vi "TF+Van der Pauw.vi"() -> ()   [LabVIEW 2022 SP3]
uses:
  <vilib>/Analysis/baseanly.llb/Mean (DBL).vi
  <vilib>/Utility/file.llb/Write Delimited Spreadsheet (DBL).vi
  <vilib>/Analysis/NI_AALBase.lvlib
panel:
  in  "FIxed F (Oe)":dbl format="%#_13g"
  out "Measured Field (Oe)":dbl=-0.24412487223744392
  out "Measured Temp (K)":dbl=2.0483396887779235
  in  "Ch2 Plot Clear":bool
  in  "Ch1 Plot Clear":bool
  out "Ch 1 phase":dbl=-151.82022434949218 caption="Ch1 phase" format="%.3p"
  out "Hall Voltage 1 phase":dbl=117.62016846841588 format="%.3p"
  out "Ch1 Current(mA)":dbl=0.0003122594054162884
  out "Hall Voltage1(mV)":dbl=0.015138421665849215
  in  "Fixed Field Approach":i32(ring) items=["Linear", "NoOvershoot", "Oscillate"]
  in  "Fixed F mode":i32(ring) items=["Persistent", "Driven"]
  in  "FIxed F Rate (Oe/s)":dbl=100.0 format="%#_13g"
  out "Hall Voltage 2 reletive phase":cluster{dbl[], dbl[]}(graph)={[0.09999999999999998, 0.12, 0.14, 0.16000000000000003, 0.17999999999999994, 0.19999999999999996, 0.21999999999999997, 0.24, 0.26, 0.28, 0.29999999999999993, 0.31999999999999995, 0.33999999999999997, 0.36, 0.38, 0.4, 0.42000000000000004, 0.43999999999999995, 0.45999999999999996, 0.48, 0.5, 0.52, 0.54, 0.56, 0.5800000000000001, 0.6, 0.62, 0.64, 0.6599999999999999, 0.6799999999999999, 0.7, 0.72, 0.74, 0.76, 0.78, 0.8, 0.8200000000000001, 0.84, 0.86, 0.88, 0.9, 0.92, 0.94, 0.96, 0.98, 1.0, 0.98, 0.96, 0.94, 0.92, 0.9, 0.88, 0.86, 0.84, 0.82, 0.8, 0.78, 0.76, 0.74, 0.72, 0.7, 0.6799999999999999, 0.66, 0.64, 0.62, 0.6, 0.58, 0.56, 0.54, 0.52, 0.5, 0.48, 0.45999999999999996, 0.44000000000000006, 0.42000000000000004, 0.4, 0.38, 0.36, 0.33999999999999997, 0.32, 0.30000000000000004, 0.28, 0.26, 0.24000000000000002, 0.22, 0.2, 0.18, 0.16, 0.14, 0.12000000000000001, 0.1, 0.09999999999999998, 0.12, 0.14, 0.16000000000000003, 0.17999999999999994, 0.19999999999999996, 0.21999999999999997, 0.24, 0.26, 0.28, 0.29999999999999993, 0.31999999999999995, 0.33999999999999997, 0.36, 0.38, 0.4, 0.42000000000000004, 0.43999999999999995, 0.45999999999999996, 0.48, 0.5, 0.52, 0.54, 0.56, 0.5800000000000001, 0.6, 0.62, 0.64, 0.6599999999999999, 0.6799999999999999, 0.7, 0.72, 0.74, 0.76, 0.78, 0.8, 0.8200000000000001, 0.84, 0.86, 0.88, 0.9, 0.92, 0.94, 0.96, 0.98, 1.0, 0.98, 0.96, 0.94, 0.92, 0.9, 0.88, 0.86, 0.84, 0.82, 0.8, 0.78, 0.76, 0.74, 0.72, 0.7, 0.6799999999999999, 0.66, 0.64, 0.62, 0.6, 0.58, 0.56, 0.54, 0.52, 0.5, 0.48, 0.45999999999999996, 0.44000000000000006, 0.42000000000000004, 0.4, 0.38, 0.36, 0.33999999999999997, 0.32, 0.30000000000000004, 0.28, 0.26, 0.24000000000000002, 0.22, 0.2, 0.18, 0.16, 0.14, 0.12000000000000001, 0.1], [117.62016846841588, 117.96664882272376, 118.35478696482726, 118.61912016643541, 118.76956664586604, 118.95054910823121, 119.01498123375443, 119.16872489157113, 119.24431424706378, 119.34190104277982, 119.41733225392822, 119.45140264855945, 119.53984114559682, 119.55691764422741, 119.59487520871042, 119.6750795139146, 119.68579169001923, 119.73065237331134, 119.74423324815396, 119.7661994334273, 119.80750346193834, 119.83623494650696, 119.82452268397942, 119.85627567058157, 119.86835371539776, 119.89360726965279, 119.90311700886441, 119.93603473890582, 119.94528450180692, 119.95000862999613, 119.95960465948625, 119.9830178122235, 119.97849406894788, 119.98959200475136, 119.99632464219606, 119.98257095958301, 120.01347012367368, 120.03103870555512, 120.04478039338926, 120.06360222149044, 120.05061637114048, 120.06363439063853, 120.07171311867637, 120.0757793318229, 120.09113199025303, 120.10726896331157, 120.06234962658894, 120.07718932923174, 120.09075423852748, 120.08476253619433, 120.05873660804704, 120.07529089338618, 120.07073006886651, 120.06602997484751, 120.06644594382928, 120.05437893498467, 120.0559832066358, 120.05241197254445, 120.03496471192462, 120.04190874507303, 120.04592984925304, 120.02590122679835, 120.02106762290221, 120.0170754772018, 120.01717601945583, 119.99024830583144, 119.98050754517847, 119.98548510957906, 119.96626810243879, 119.94421874372571, 119.91496186190318, 119.90254071057821, 119.89802448935203, 119.86225587700838, 119.84782030921231, 119.76071599522875, 119.78171218684165, 119.52712081973637, 119.68947818038498, 119.64888776868774, 119.54538024283588, 119.49187757183782, 119.40373568864177, 119.34094898550048, 119.25703379849283, 119.03268380413638, 118.93848534047406, 118.66368000738926, 118.3703709122756, 118.00894457485364, 117.8022869674905, 117.83191820734878, 118.35839994290589, 118.74306406859516, 118.97978381368443, 119.0832443256442, 119.22408053378842, 119.3756798875886, 119.42654507577663, 119.54312088447948, 119.65528936579355, 119.68067384348709, 119.73888591320637, 119.7746550722424, 119.83575660206921, 119.87436287491752, 119.92090575023776, 119.96360858392154, 119.97618916031327, 120.0270490763764, 120.03660757353578, 120.04594971613244, 120.07374861282088, 120.08502945701846, 120.11904718233538, 120.12373738373853, 120.13187955586031, 120.15078785675374, 120.16051712055169, 120.18138633972099, 120.18855573342282, 120.20283710115059, 120.21752926335739, 120.2286670939815, 120.25005622275296, 120.26083012867937, 120.26435687292016, 120.25219743715516, 120.27247788976976, 120.27728128431886, 120.30980987455453, 120.3013104315504, 120.30956542774932, 120.32575192936613, 120.32481345899741, 120.34376176879596, 120.32045496743885, 120.31980339045367, 120.31350527912403, 120.31252525198906, 120.3242014431218, 120.34462619894298, 120.32098729633576, 120.3242809008918, 120.31759933903815, 120.34279447419958, 120.29133105012681, 120.2971043007052, 120.2915107827317, 120.30887402170481, 120.3132908103599, 120.29180381456831, 120.29677581115975, 120.25488350003204, 120.25012405536286, 120.24749071884021, 120.20434065293489, 120.23689420155657, 120.20258149493482, 120.19465503125453, 120.16140368284456, 120.17158365673114, 120.12877813062116, 120.10707856478476, 120.07296661494834, 120.03335070293379, 120.02574871514983, 119.97110769112416, 120.18824358128647, 119.87610802993717, 119.85772779265321, 119.77209829112437, 119.73583766352138, 119.65849570448214, 119.57056721383769, 119.43100181965622, 119.2628284467831, 119.0562851102115, 118.80762144883226, 118.56712932086603, 117.71722366335914, 116.41351313841975, 116.41351313841975]}
  out "Hall Voltage 1 reletive phase":cluster{dbl[], dbl[]}(graph)={[0.09999999999999998, 0.12, 0.14, 0.16000000000000003, 0.17999999999999994, 0.19999999999999996, 0.21999999999999997, 0.24, 0.26, 0.28, 0.29999999999999993, 0.31999999999999995, 0.33999999999999997, 0.36, 0.38, 0.4, 0.42000000000000004, 0.43999999999999995, 0.45999999999999996, 0.48, 0.5, 0.52, 0.54, 0.56, 0.5800000000000001, 0.6, 0.62, 0.64, 0.6599999999999999, 0.6799999999999999, 0.7, 0.72, 0.74, 0.76, 0.78, 0.8, 0.8200000000000001, 0.84, 0.86, 0.88, 0.9, 0.92, 0.94, 0.96, 0.98, 1.0, 0.98, 0.96, 0.94, 0.92, 0.9, 0.88, 0.86, 0.84, 0.82, 0.8, 0.78, 0.76, 0.74, 0.72, 0.7, 0.6799999999999999, 0.66, 0.64, 0.62, 0.6, 0.58, 0.56, 0.54, 0.52, 0.5, 0.48, 0.45999999999999996, 0.44000000000000006, 0.42000000000000004, 0.4, 0.38, 0.36, 0.33999999999999997, 0.32, 0.30000000000000004, 0.28, 0.26, 0.24000000000000002, 0.22, 0.2, 0.18, 0.16, 0.14, 0.12000000000000001, 0.1, 0.09999999999999998, 0.12, 0.14, 0.16000000000000003, 0.17999999999999994, 0.19999999999999996, 0.21999999999999997, 0.24, 0.26, 0.28, 0.29999999999999993, 0.31999999999999995, 0.33999999999999997, 0.36, 0.38, 0.4, 0.42000000000000004, 0.43999999999999995, 0.45999999999999996, 0.48, 0.5, 0.52, 0.54, 0.56, 0.5800000000000001, 0.6, 0.62, 0.64, 0.6599999999999999, 0.6799999999999999, 0.7, 0.72, 0.74, 0.76, 0.78, 0.8, 0.8200000000000001, 0.84, 0.86, 0.88, 0.9, 0.92, 0.94, 0.96, 0.98, 1.0, 0.98, 0.96, 0.94, 0.92, 0.9, 0.88, 0.86, 0.84, 0.82, 0.8, 0.78, 0.76, 0.74, 0.72, 0.7, 0.6799999999999999, 0.66, 0.64, 0.62, 0.6, 0.58, 0.56, 0.54, 0.52, 0.5, 0.48, 0.45999999999999996, 0.44000000000000006, 0.42000000000000004, 0.4, 0.38, 0.36, 0.33999999999999997, 0.32, 0.30000000000000004, 0.28, 0.26, 0.24000000000000002, 0.22, 0.2, 0.18, 0.16, 0.14, 0.12000000000000001, 0.1], [-151.82022434949218, -151.31250474861076, -150.934829382567, -150.48587961112963, -150.35129794100732, -150.20108675684463, -150.07301012387398, -149.85371662190408, -149.80643007097768, -149.6778115966004, -149.70631232196195, -149.3427081876464, -144.00790971737905, -149.75303510022803, -149.67465048111166, -149.61059645892314, -149.5755216627079, -149.56032591732512, -149.56777135196236, -149.53038555798872, -149.4837567137922, -149.46653630858634, -149.4555130589029, -149.44977309701568, -149.46602213201024, -149.42050625632652, -149.44267585686146, -149.44000832559337, -149.42583379539636, -149.39692572431568, -149.40442155131146, -149.40915566881102, -149.38050614114596, -149.38240574949845, -149.3953243906204, -149.3899047221218, -149.38685008550175, -149.37072119411883, -149.37324923858517, -149.36914979835484, -149.37390639605138, -149.3980165878626, -149.38623806135408, -149.35518531108906, -149.37819742529774, -149.37025076997705, -149.37797439572273, -149.4274062049048, -149.39553532551332, -149.39989159256442, -149.40788326839706, -149.4035269042052, -149.42173829217444, -149.42516481564763, -149.4219167404996, -149.46356168834444, -149.4516805103338, -149.45047160544362, -149.45716135037998, -149.47450752769095, -149.4832252279336, -149.49183740199788, -149.51226639630787, -149.525555046651, -149.5573781565128, -149.5590093788641, -149.5858478680793, -149.5557150450339, -149.61888489114702, -149.65084954099694, -149.65437010384474, -149.69488018826033, -149.69116543387327, -149.7564704385459, -149.77576215560174, -149.78827998741025, -150.21783070990878, -156.94726445856756, -149.75208834187845, -149.79358735688876, -149.81920487838278, -149.97644416993913, -150.0531791626578, -150.16748042818656, -150.30076394633943, -150.44483707228213, -150.66626270081673, -151.04929447184827, -151.43411807203063, -151.97278023054187, -152.18821211537258, -152.14623356637654, -151.4719825276092, -150.96302427747355, -150.84756504567386, -150.5037700822142, -150.3245640418613, -150.17713325364664, -150.1036649225191, -149.99036753477975, -149.85697295444248, -149.8501754093205, -149.56080314237312, -146.67158122655187, -149.96749106410877, -149.93190810259412, -149.9232306144384, -149.8834345316244, -149.82170489643204, -149.7789775276986, -149.77872756893103, -149.7707527140453, -149.75157225999848, -149.7012296966859, -149.71638923850873, -149.69938903054089, -149.67312320269653, -149.69041977164406, -149.6838198853977, -149.66161778220618, -149.6546278866485, -149.640923821836, -149.6728863842432, -149.66791865505627, -149.62858582517933, -149.64183587402476, -149.6484558455101, -149.6427424788427, -149.6296817347956, -149.63395082883616, -149.62713187401155, -149.6182616601406, -149.65041315650092, -149.62494744989198, -149.61909696518853, -149.6175044512262, -149.6371509732279, -149.66137383135944, -149.63515614075328, -149.6451064613961, -149.65811060587708, -149.64909805431552, -149.6696824809014, -149.66829454461902, -149.65211834334818, -149.6792564836343, -149.69346020858046, -149.7169451406854, -149.71160254963883, -149.72665337378038, -149.73853617494782, -149.73020826238755, -149.75385526179556, -149.7724664962522, -149.77034769159013, -149.80481526391884, -149.81816596924764, -149.87205062927146, -149.86012342940273, -149.90891882509268, -149.92420949696478, -149.94160073513336, -149.98031714888242, -149.98297286567293, -150.01739729399605, -150.0978801191893, -150.09675943096, -149.9722562160305, -148.8947110005267, -150.0746278787694, -150.12829367372765, -150.21097166683603, -150.2349660580826, -150.3575760488762, -150.49529547074826, -150.72432289368865, -150.81632873807234, -151.05780214090098, -151.3722097867961, -151.68469888569936, -152.04933901054727, -152.04933901054727]}
  out "Hall Voltage 2":cluster{dbl[], dbl[]}(graph)={[0.09999999999999998, 0.12, 0.14, 0.16000000000000003, 0.17999999999999994, 0.19999999999999996, 0.21999999999999997, 0.24, 0.26, 0.28, 0.29999999999999993, 0.31999999999999995, 0.33999999999999997, 0.36, 0.38, 0.4, 0.42000000000000004, 0.43999999999999995, 0.45999999999999996, 0.48, 0.5, 0.52, 0.54, 0.56, 0.5800000000000001, 0.6, 0.62, 0.64, 0.6599999999999999, 0.6799999999999999, 0.7, 0.72, 0.74, 0.76, 0.78, 0.8, 0.8200000000000001, 0.84, 0.86, 0.88, 0.9, 0.92, 0.94, 0.96, 0.98, 1.0, 0.98, 0.96, 0.94, 0.92, 0.9, 0.88, 0.86, 0.84, 0.82, 0.8, 0.78, 0.76, 0.74, 0.72, 0.7, 0.6799999999999999, 0.66, 0.64, 0.62, 0.6, 0.58, 0.56, 0.54, 0.52, 0.5, 0.48, 0.45999999999999996, 0.44000000000000006, 0.42000000000000004, 0.4, 0.38, 0.36, 0.33999999999999997, 0.32, 0.30000000000000004, 0.28, 0.26, 0.24000000000000002, 0.22, 0.2, 0.18, 0.16, 0.14, 0.12000000000000001, 0.1, 0.09999999999999998, 0.12, 0.14, 0.16000000000000003, 0.17999999999999994, 0.19999999999999996, 0.21999999999999997, 0.24, 0.26, 0.28, 0.29999999999999993, 0.31999999999999995, 0.33999999999999997, 0.36, 0.38, 0.4, 0.42000000000000004, 0.43999999999999995, 0.45999999999999996, 0.48, 0.5, 0.52, 0.54, 0.56, 0.5800000000000001, 0.6, 0.62, 0.64, 0.6599999999999999, 0.6799999999999999, 0.7, 0.72, 0.74, 0.76, 0.78, 0.8, 0.8200000000000001, 0.84, 0.86, 0.88, 0.9, 0.92, 0.94, 0.96, 0.98, 1.0, 0.98, 0.96, 0.94, 0.92, 0.9, 0.88, 0.86, 0.84, 0.82, 0.8, 0.78, 0.76, 0.74, 0.72, 0.7, 0.6799999999999999, 0.66, 0.64, 0.62, 0.6, 0.58, 0.56, 0.54, 0.52, 0.5, 0.48, 0.45999999999999996, 0.44000000000000006, 0.42000000000000004, 0.4, 0.38, 0.36, 0.33999999999999997, 0.32, 0.30000000000000004, 0.28, 0.26, 0.24000000000000002, 0.22, 0.2, 0.18, 0.16, 0.14, 0.12000000000000001, 0.1], [12.205176752147196, 12.33738736524411, 12.436814472113113, 12.543061919618381, 12.591177109870843, 12.63204488402351, 12.633074379656962, 12.678587031476285, 12.702366812156168, 12.734766256641889, 12.764822745445459, 12.798115074151369, 12.56005416503157, 12.811022273559901, 12.805614848037402, 12.822742652741233, 12.833360063934796, 12.844414076677566, 12.853037374725659, 12.863749846343488, 12.873727971040198, 12.87545677652524, 12.884395543563812, 12.901595012846315, 12.91020558633629, 12.91700210310611, 12.916182386400777, 12.932745625307929, 12.929132177243485, 12.939245398543807, 12.945904132779514, 12.979271768015096, 12.951619927398129, 12.963100847085817, 12.961454764152798, 12.968676853276186, 13.035314574413999, 12.968769140450755, 12.976857768700619, 12.982937075765706, 12.987156955464599, 12.987225357622929, 12.990469558247861, 13.001074140628084, 13.015805070701896, 13.213316441028162, 13.212674850256546, 13.214497097772925, 13.213097914485022, 13.212520778890907, 13.217287379489568, 13.224571659209413, 13.221461422183241, 13.21249046212996, 13.231625931101464, 13.219596872719654, 13.230780717880945, 13.231496283261466, 13.228879184378412, 13.236537684484286, 13.2442021665191, 13.245327395573094, 13.239075527873267, 13.250459225400578, 13.254010022147359, 13.263592058540043, 13.278201777756056, 13.271280645160415, 13.28286228675346, 13.287261154844275, 13.290082368268422, 13.30492697157085, 13.325287026560359, 13.337097306813405, 13.334459335710374, 13.36121908059594, 13.349781951942722, 13.590657500379482, 13.420711749521754, 13.427055186068772, 13.476488972924022, 13.504746276159453, 13.521802810703734, 13.585085247505193, 13.63738342595085, 13.703337851038048, 13.791442558469074, 13.849252925446702, 13.98837153260088, 14.058767459755813, 13.057484778983863, 12.424975150602982, 12.341214474536581, 12.597671651852279, 12.547100753140823, 12.603242737801498, 12.610091337495355, 12.662729976248402, 12.683644441406994, 12.707706571670649, 12.74751634316906, 12.764099115085513, 12.803871979165852, 12.693242845243883, 12.809727121728208, 12.817180050708686, 12.831651755770647, 12.839364718018068, 12.860298160932963, 12.896827552552299, 12.864701328486037, 12.883685199780242, 12.884793998467885, 12.902011985965638, 12.898401964032054, 12.906219259474547, 12.914228868687658, 12.911587003388147, 12.958793693981802, 12.933506906195795, 12.933859306721546, 12.94206688909155, 12.946106387292451, 12.954120795402451, 12.95420497189929, 12.961692049093307, 12.970243175218398, 12.966251377610806, 12.971030269555348, 12.980713661496962, 12.983816343381182, 12.98792173316417, 12.995117688102317, 13.000724459135895, 13.003773018187172, 13.013804312695264, 13.221409487304983, 13.213732944734987, 13.219930146403511, 13.2160660705417, 13.220288758106749, 13.225356431589839, 13.221627768983318, 13.192042140412925, 13.225457206093656, 13.224404733921627, 13.226943621029603, 13.22188486286242, 13.239906219746997, 13.23627215525837, 13.23780083001927, 13.24191338088606, 13.243188029364342, 13.248586751116793, 13.24553444444596, 13.263702564618967, 13.263180218458823, 13.265510887371871, 13.27580985473867, 13.285902114226138, 13.285290341366075, 13.292004389335341, 13.320520276023231, 13.32468083832859, 13.320587416172566, 13.3596713753944, 13.351640175534053, 13.311511157505569, 13.749204463952886, 13.417895997650705, 13.439008654275602, 13.464312581366862, 13.491545253041302, 13.546146393015691, 13.560171412898399, 13.584913714835219, 13.647701856221694, 13.605003489243288, 13.892818025978201, 13.94644999851722, 14.42599048649726, 102.36268705136854, 102.36268705136854]}
  out "Hall Voltage 1":cluster{dbl[], dbl[]}(graph)={[0.09999999999999998, 0.12, 0.14, 0.16000000000000003, 0.17999999999999994, 0.19999999999999996, 0.21999999999999997, 0.24, 0.26, 0.28, 0.29999999999999993, 0.31999999999999995, 0.33999999999999997, 0.36, 0.38, 0.4, 0.42000000000000004, 0.43999999999999995, 0.45999999999999996, 0.48, 0.5, 0.52, 0.54, 0.56, 0.5800000000000001, 0.6, 0.62, 0.64, 0.6599999999999999, 0.6799999999999999, 0.7, 0.72, 0.74, 0.76, 0.78, 0.8, 0.8200000000000001, 0.84, 0.86, 0.88, 0.9, 0.92, 0.94, 0.96, 0.98, 1.0, 0.98, 0.96, 0.94, 0.92, 0.9, 0.88, 0.86, 0.84, 0.82, 0.8, 0.78, 0.76, 0.74, 0.72, 0.7, 0.6799999999999999, 0.66, 0.64, 0.62, 0.6, 0.58, 0.56, 0.54, 0.52, 0.5, 0.48, 0.45999999999999996, 0.44000000000000006, 0.42000000000000004, 0.4, 0.38, 0.36, 0.33999999999999997, 0.32, 0.30000000000000004, 0.28, 0.26, 0.24000000000000002, 0.22, 0.2, 0.18, 0.16, 0.14, 0.12000000000000001, 0.1, 0.09999999999999998, 0.12, 0.14, 0.16000000000000003, 0.17999999999999994, 0.19999999999999996, 0.21999999999999997, 0.24, 0.26, 0.28, 0.29999999999999993, 0.31999999999999995, 0.33999999999999997, 0.36, 0.38, 0.4, 0.42000000000000004, 0.43999999999999995, 0.45999999999999996, 0.48, 0.5, 0.52, 0.54, 0.56, 0.5800000000000001, 0.6, 0.62, 0.64, 0.6599999999999999, 0.6799999999999999, 0.7, 0.72, 0.74, 0.76, 0.78, 0.8, 0.8200000000000001, 0.84, 0.86, 0.88, 0.9, 0.92, 0.94, 0.96, 0.98, 1.0, 0.98, 0.96, 0.94, 0.92, 0.9, 0.88, 0.86, 0.84, 0.82, 0.8, 0.78, 0.76, 0.74, 0.72, 0.7, 0.6799999999999999, 0.66, 0.64, 0.62, 0.6, 0.58, 0.56, 0.54, 0.52, 0.5, 0.48, 0.45999999999999996, 0.44000000000000006, 0.42000000000000004, 0.4, 0.38, 0.36, 0.33999999999999997, 0.32, 0.30000000000000004, 0.28, 0.26, 0.24000000000000002, 0.22, 0.2, 0.18, 0.16, 0.14, 0.12000000000000001, 0.1], [2087.542522514706, 2143.3806726181297, 2192.1505680332307, 2224.5398110134415, 2254.2076727564463, 2283.219391571736, 2295.5351896243988, 2312.274969759326, 2321.1906487058636, 2258.618428233254, 2439.815278150036, 2363.114732601407, 2569.2987357483867, 2366.69462809311, 2370.3526096767628, 2370.7532832147513, 2369.446453774161, 2372.3479615014453, 2373.7967150363133, 2373.3912011059742, 2374.3898629584414, 2373.19922105906, 2374.08711510194, 2374.3447992304204, 2372.719181172187, 2372.5831623830313, 2368.606666524962, 2368.1271954116123, 2368.1587157781582, 2368.364263936688, 2363.1239774166042, 2363.4322755470225, 2359.5286066627255, 2362.2730811990377, 2355.540999658394, 2354.6901938211345, 2338.3987997031136, 2348.956030561271, 2348.6720464600826, 2345.47931492513, 2343.641628918994, 2322.579102266805, 2357.7528780540633, 2337.9624461876765, 2337.035655864342, 2390.13340514578, 2393.333076080936, 2397.194891434832, 2400.4646152722025, 2404.1840381335187, 2406.4647119031993, 2411.655350773428, 2414.452737749684, 2416.491207784975, 2422.152414810807, 2426.43445652573, 2430.4661399145198, 2472.9095612064084, 2401.2074203638863, 2442.381915486605, 2447.39053615182, 2448.9505311169605, 2454.873847352734, 2458.903517524707, 2461.995925756737, 2467.061840825975, 2470.520942891029, 2474.931087852616, 2483.997180170197, 2486.4806066909064, 2489.8094006815363, 2495.4829515630936, 2496.5109281850623, 2499.717712613259, 2508.0628602511415, 2587.583625405099, 2446.457085912187, 2744.1467541037973, 2527.145831911331, 2528.3781519262234, 2531.0945072462814, 2536.7135748602786, 2544.038687449601, 2544.827299932163, 2546.39588450735, 2552.3831526464273, 2560.7487646591876, 2557.6068386083666, 2541.8036010528517, 2556.5211525031086, 2275.4515181505535, 2236.3211050589766, 2137.0989873521185, 2148.4934229155265, 2226.3795783020046, 2259.8236048661397, 2277.518588977397, 2298.2309636749364, 2311.745843167506, 2328.4510173480307, 2336.560722824512, 2344.24126014681, 2362.7311144000346, 2627.003456834187, 2364.144130172327, 2369.8717620699094, 2373.0451002371196, 2373.971931289017, 2377.1037991880976, 2381.4533155017552, 2376.2465418035545, 2376.4643282086604, 2373.1094722464964, 2373.683408097068, 2373.6902390420423, 2372.436584742077, 2372.7068819175765, 2370.444178339574, 2369.7303118006134, 2368.9013786355426, 2364.66910807676, 2363.1277468576277, 2362.1693752579, 2359.8572707523836, 2358.3637082703754, 2356.2088803095526, 2354.2381091107436, 2352.2504633571566, 2349.807036392201, 2348.000550307495, 2345.2605399911095, 2343.048947126772, 2342.138893566093, 2338.647207375316, 2337.823575605664, 2336.4325858086618, 2391.3050818760403, 2393.854078139158, 2397.3144621611436, 2400.183701016868, 2404.559873121706, 2408.113986664911, 2411.3881576090257, 2422.2503149813315, 2418.4477629937755, 2423.424584031643, 2427.359469208306, 2429.5536317154106, 2435.189541439222, 2439.3273653599067, 2443.6532125172207, 2446.4799477219917, 2450.5183688798943, 2455.1086830020786, 2469.17017360265, 2463.7910814680667, 2466.142256138314, 2475.164122601692, 2480.58039686262, 2485.3434347885513, 2489.254932267259, 2490.995762828881, 2496.288772114335, 2501.89872487851, 2502.665922214194, 2507.8176213420734, 2510.8951882690485, 2514.6646388029453, 2515.90870103181, 2526.343933365244, 2527.8233287119538, 2535.9588766433053, 2534.614384395244, 2541.4565246972834, 2550.357749348691, 2549.473660870641, 2558.3365999756966, 2604.730472408435, 2561.1991565610233, 2554.929997465301, 2611.611284193903, 2611.611284193903]}
  out "Hall Voltage 2 phase":dbl=117.62016846841588 format="%.3p"
  out "Ch 2 phase":dbl=-151.82022434949218 caption="Ch2 phase" format="%.3p"
  out "Hall Voltage2(mV)":dbl=0.015138421665849215
  out "Ch2 Current(mA)":dbl=0.0003122594054162884
  in  "R2(Kohm)":dbl=1.9997 format="%#_13g"
  in  "R1(Kohm)":dbl=2.0265 format="%#_13g"
  in  "path2 (folder + filename)":string="G:\\My Drive\\Opticool\\Measurement\\NLH\\T dependence\\TaI28_A1215_B1211"
  in  "Save data or not":bool=TRUE
  in  "path1 (folder + filename)":string="G:\\My Drive\\Opticool\\Measurement\\NLH\\T dependence\\TaI27_A34_B38"
  in  "V Loop#":i32=1
  in  "Two Channels ?":bool=TRUE
  in  "LOCKIN2 address":refnum<visa-resource-name>="COM4"
  in  "2B frequency 2":dbl=26.7 format="%#_13g"
  in  "2B Input Connection (0: Single-Ended)":u16(ring)=1 items=["Single-Ended Voltage", "Differential Voltage", "1 MOhm Current Gain", "100 MOhm Current Gain"]
  in  "2B harmonic 1":u8=2
  in  "2B harmonic 2":u8=3
  in  "2B reference Manual Phase":dbl
  in  "auto phase 2B":bool=TRUE
  in  "2B Sample time (s)":dbl=0.001 min=0.001 max=100.0 step=0.001
  in  "2B Sensitivity":u16(ring)=26 items=["1 nV/fA", "2 nV/fA", "5 nV/fA", "10 nV/fA", "20 nV/fA", "50 nV/fA", "100 nV/fA", "200 nV/fA", "500 nV/fA", "1 uV/pA", "2 uV/pA", "5 uV/pA", "10 uV/pA", "20 uV/pA", "50 uV/pA", "100 uV/pA", "200 uV/pA", "500 uV/pA", "1 mV/nA", "2 mV/nA", "5 mV/nA", "10 mV/nA", "20 mV/nA", "50 mV/nA", "100 mV/nA", "200 mV/nA", "500 mV/nA", "1 V/uA"]
  in  "Enable Sync Filter 2B (open when f<200Hz)":bool
  in  "2B Time Constant":u8(ring)=9 items=["10 us", "30 us", "100 us", "300 us", "1 ms", "3 ms", "10 ms", "30 ms", "100 ms", "300 ms", "1 s", "3 s", "10 s", "30 s", "100 s", "300 s", "1 ks", "3 ks"]
  in  "2B Reference Source":u8(ring)=3 items=["External", "Internal", "Internal Sweep", "Channel-A"]
  in  "2B Low Pass Filter Slope":u8(ring)=2 items=["6 dB/oct", "12 dB/oct", "18 db/oct", "24 dB/oct"]
  in  "2A frequency":dbl=16.7 format="%#_13g"
  in  "2A Input Connection (0: Single-Ended)":u16(ring)=1 items=["Single-Ended Voltage", "Differential Voltage", "1 MOhm Current Gain", "100 MOhm Current Gain"]
  in  "2A harmonic 1":u8=2
  in  "2A harmonic 2":u8=3
  in  "2A reference Manual Phase":dbl
  in  "auto phase 2A":bool=TRUE
  in  "2A Reference Source":u8(ring)=1 items=["External", "Internal", "Internal Sweep"]
  in  "2A Sample time (s)":dbl=0.001 min=0.001 max=100.0 step=0.001
  in  "2A Time Constant":u8(ring)=9 items=["10 us", "30 us", "100 us", "300 us", "1 ms", "3 ms", "10 ms", "30 ms", "100 ms", "300 ms", "1 s", "3 s", "10 s", "30 s", "100 s", "300 s", "1 ks", "3 ks"]
  in  "Enable Sync Filter 2A (open when f<200Hz)":bool
  in  "2A Sensitivity":u16(ring)=26 items=["1 nV/fA", "2 nV/fA", "5 nV/fA", "10 nV/fA", "20 nV/fA", "50 nV/fA", "100 nV/fA", "200 nV/fA", "500 nV/fA", "1 uV/pA", "2 uV/pA", "5 uV/pA", "10 uV/pA", "20 uV/pA", "50 uV/pA", "100 uV/pA", "200 uV/pA", "500 uV/pA", "1 mV/nA", "2 mV/nA", "5 mV/nA", "10 mV/nA", "20 mV/nA", "50 mV/nA", "100 mV/nA", "200 mV/nA", "500 mV/nA", "1 V/uA"]
  in  "2A Low Pass Filter Slope":u8(ring)=2 items=["6 dB/oct", "12 dB/oct", "18 db/oct", "24 dB/oct"]
  in  "T Delay":dbl=1500.0
  out "Temperature":dbl
  out "Field":dbl
  out "Field Status":i32(ring) items=["MagnetUnknown"=0, "StablePersistent"=1, "WarmingSwitch"=2, "CoolingSwitch"=3, "StableDriven"=4, "Iterating"=5, "Charging"=6, "Discharging"=7, "CurrentError"=8, "MagnetFailure"=15]
  out "Temperature Status":i32(ring) items=["TemperatureUnknown"=0, "Stable"=1, "Tracking"=2, "Near"=5, "Chasing"=6, "Filling"=7, "Standby"=10, "Disabled"=13, "ImpedanceNotFunction"=14, "TempFailure"=15]
  in  "?":bool
  out "Sine voltage T":dbl=0.09999999999999998 format="%#_13g"
  in  "Initialization?":bool
  in  "F Delay":dbl=5.0
  out "Backward":bool
  out "Forward":bool=TRUE
  in  "V Step(mV)":i32=100
  out "V Loop Run T":i32=1
  in  "High Value (V)":dbl=3.0
  in  "Low Value (V)":dbl=0.1
  in  "System Stablization (s)":dbl=0.5 format="%#_13g"
  in  "Sweep Temperature Approach":i32(ring)=1 items=["FastSettle", "NoOvershoot"]
  in  "Sweep T  Rate (K/min)":dbl=10.0
  in  "Remote":bool=TRUE
  in  "IP Address":string="169.254.170.239"
  out "Measuring":bool
  in  "LOCKIN1 address":refnum<visa-resource-name>="COM3"
  out "Temp Setting":dbl=2.0 format="%#_13g"
  in  "Step(K)":i32=10
  in  "B frequency":dbl=26.7 format="%#_13g"
  in  "B Input Connection (0: Single-Ended)":u16(ring)=1 items=["Single-Ended Voltage", "Differential Voltage", "1 MOhm Current Gain", "100 MOhm Current Gain"]
  in  "B harmonic 1":u8=2
  in  "B harmonic 2":u8=3
  in  "B reference Manual Phase":dbl
  in  "auto phase B":bool=TRUE
  in  "B Sample time (s)":dbl=0.001 min=0.001 max=100.0 step=0.001
  in  "B Sensitivity":u16(ring)=26 items=["1 nV/fA", "2 nV/fA", "5 nV/fA", "10 nV/fA", "20 nV/fA", "50 nV/fA", "100 nV/fA", "200 nV/fA", "500 nV/fA", "1 uV/pA", "2 uV/pA", "5 uV/pA", "10 uV/pA", "20 uV/pA", "50 uV/pA", "100 uV/pA", "200 uV/pA", "500 uV/pA", "1 mV/nA", "2 mV/nA", "5 mV/nA", "10 mV/nA", "20 mV/nA", "50 mV/nA", "100 mV/nA", "200 mV/nA", "500 mV/nA", "1 V/uA"]
  in  "Enable Sync Filter B (open when f<200Hz)":bool
  in  "B Time Constant":u8(ring)=9 items=["10 us", "30 us", "100 us", "300 us", "1 ms", "3 ms", "10 ms", "30 ms", "100 ms", "300 ms", "1 s", "3 s", "10 s", "30 s", "100 s", "300 s", "1 ks", "3 ks"]
  in  "B Reference Source":u8(ring)=3 items=["External", "Internal", "Internal Sweep", "Channel-A"]
  in  "B Low Pass Filter Slope":u8(ring)=2 items=["6 dB/oct", "12 dB/oct", "18 db/oct", "24 dB/oct"]
  in  "A frequency":dbl=26.7 format="%#_13g"
  in  "A Input Connection (0: Single-Ended)":u16(ring)=1 items=["Single-Ended Voltage", "Differential Voltage", "1 MOhm Current Gain", "100 MOhm Current Gain"]
  in  "A harmonic 1":u8=2
  in  "A harmonic 2":u8=3
  in  "A reference Manual Phase":dbl
  in  "auto phase A":bool=TRUE
  in  "A Reference Source":u8(ring)=1 items=["External", "Internal", "Internal Sweep"]
  in  "A Sample time (s)":dbl=0.001 min=0.001 max=100.0 step=0.001
  in  "A Time Constant":u8(ring)=9 items=["10 us", "30 us", "100 us", "300 us", "1 ms", "3 ms", "10 ms", "30 ms", "100 ms", "300 ms", "1 s", "3 s", "10 s", "30 s", "100 s", "300 s", "1 ks", "3 ks"]
  in  "Enable Sync Filter A (open when f<200Hz)":bool
  in  "A Sensitivity":u16(ring)=26 items=["1 nV/fA", "2 nV/fA", "5 nV/fA", "10 nV/fA", "20 nV/fA", "50 nV/fA", "100 nV/fA", "200 nV/fA", "500 nV/fA", "1 uV/pA", "2 uV/pA", "5 uV/pA", "10 uV/pA", "20 uV/pA", "50 uV/pA", "100 uV/pA", "200 uV/pA", "500 uV/pA", "1 mV/nA", "2 mV/nA", "5 mV/nA", "10 mV/nA", "20 mV/nA", "50 mV/nA", "100 mV/nA", "200 mV/nA", "500 mV/nA", "1 V/uA"]
  in  "A Low Pass Filter Slope":u8(ring)=2 items=["6 dB/oct", "12 dB/oct", "18 db/oct", "24 dB/oct"]
  in  "End Value (K)":dbl=302.0
  in  "Start Value (K)":dbl=2.0
  in  "Single/Double":i32=1 min=1 max=2 step=1
  # "Statue"
  # "Ch1 Measurement"
  # "Lock-in Setting"
  # "Channel 1A"
  # "Sweep Setting"
  # "Channel 1B"
  # "Channel 2A"
  # "Current Measurement"
  # "Channel 2B"
  # "Ch2 Measurement"
  # "Temprature and Field Setting"
  # "Sweep T"
  # "F Setting"
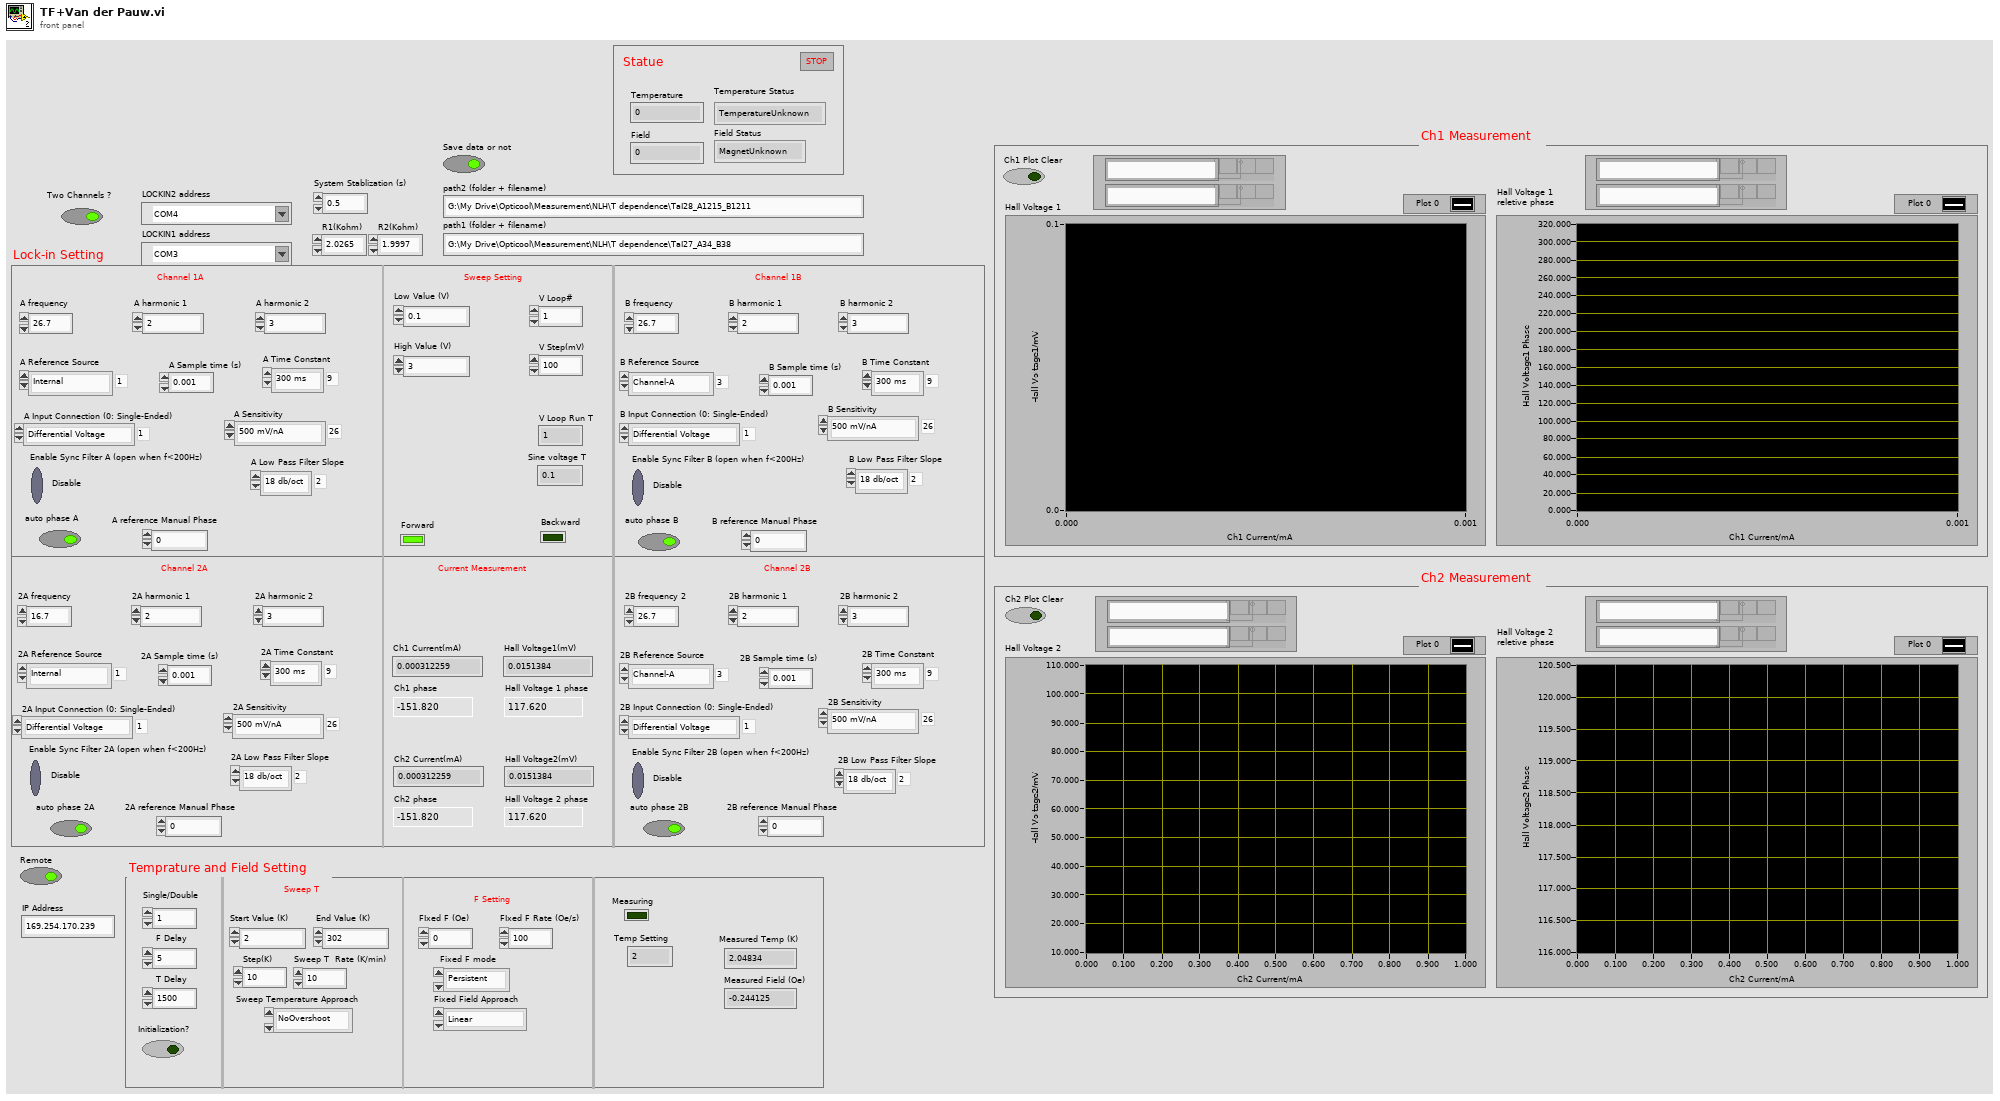
[diagram p1: front panel]
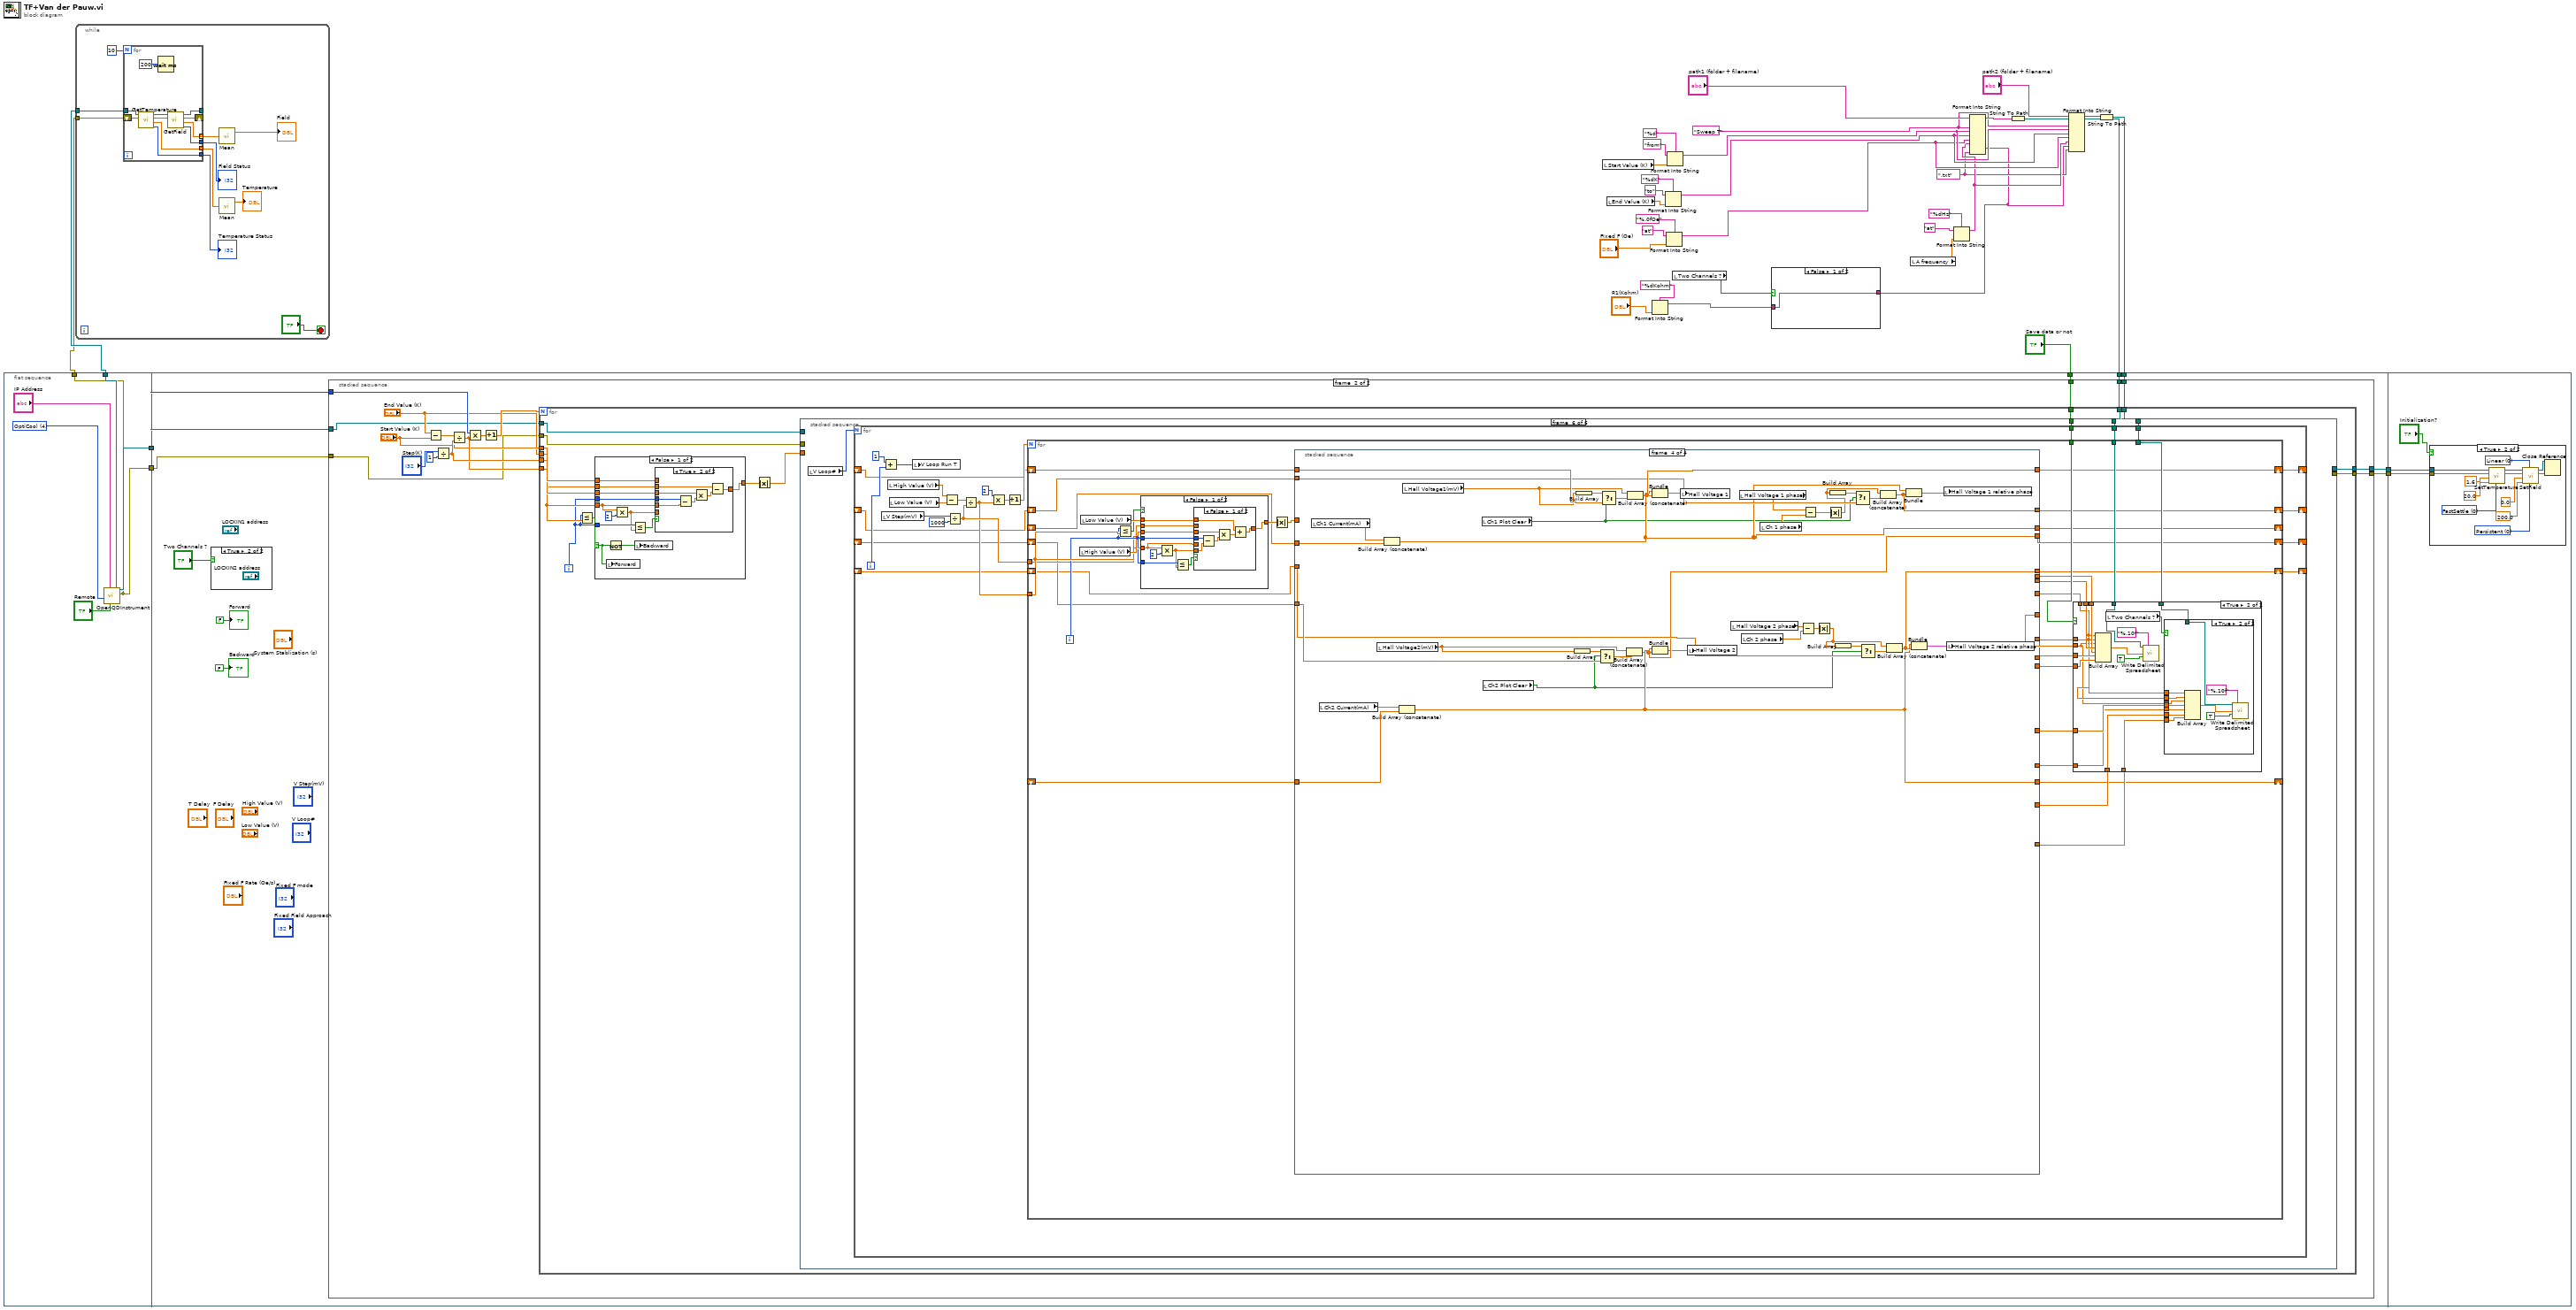
[diagram p0: block diagram]
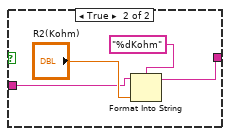
[diagram p2: hidden frame]
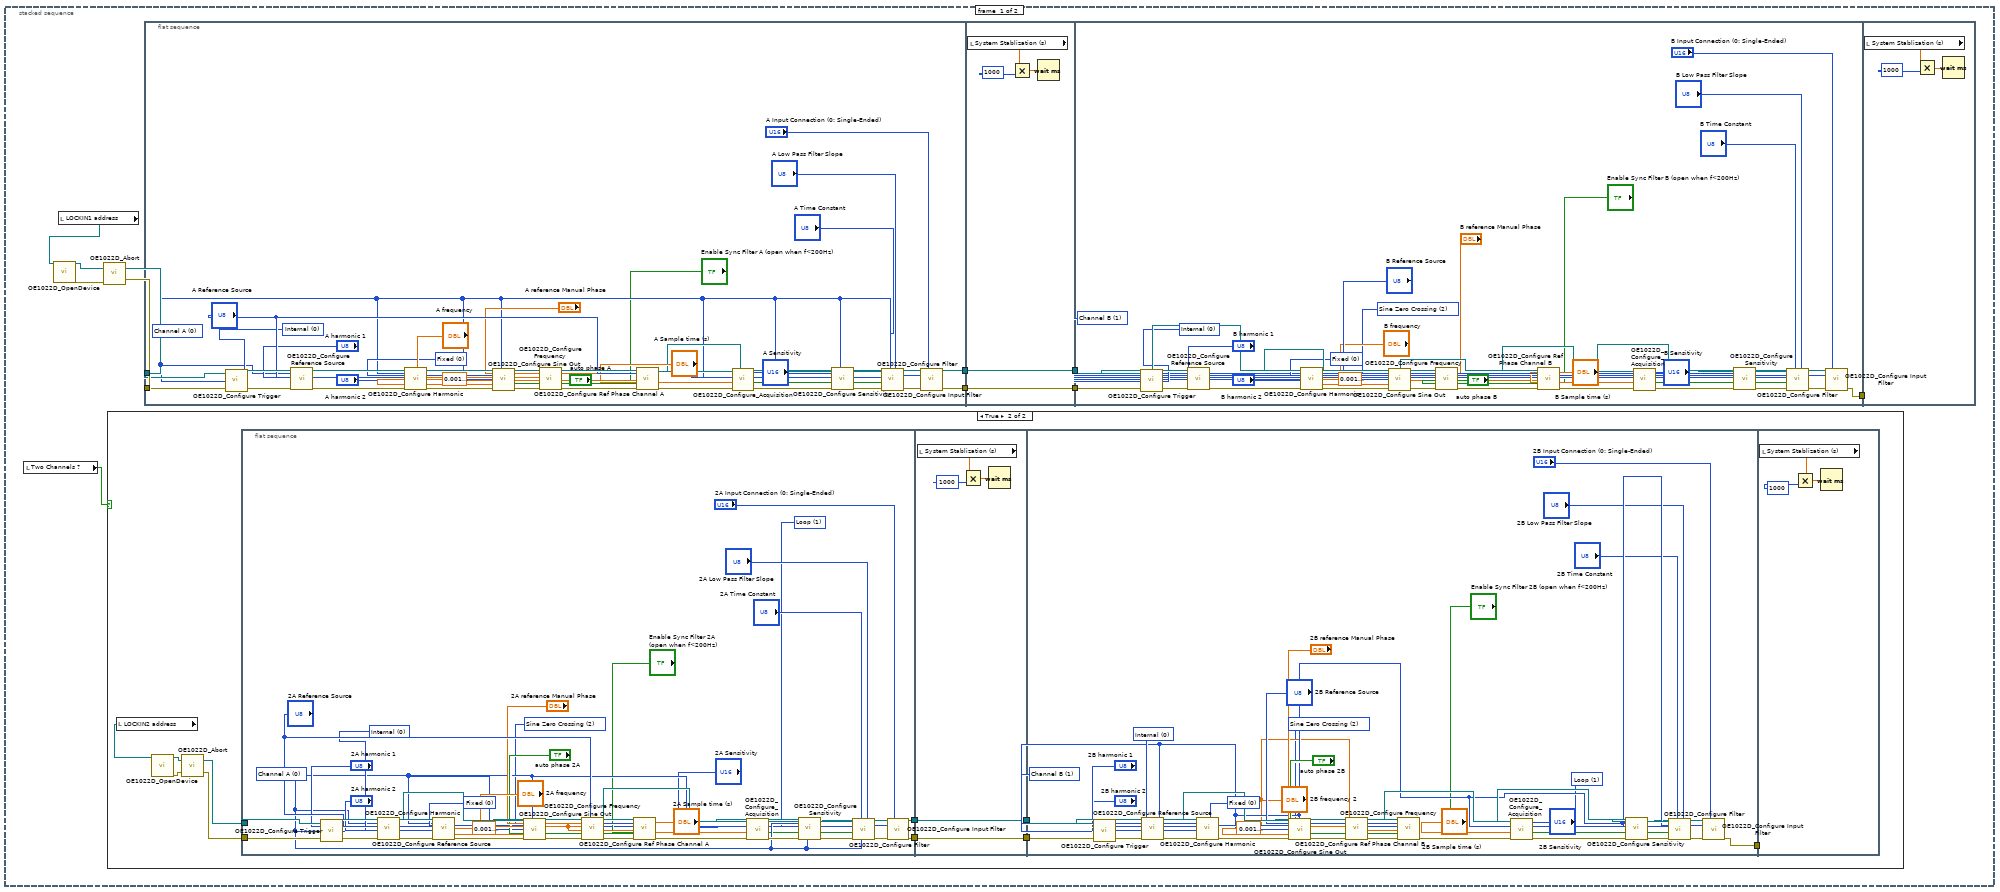
[diagram p4: hidden frame]
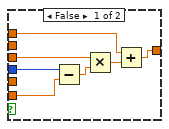
[diagram p6: hidden frame]
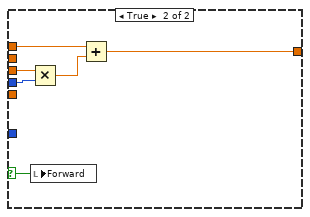
[diagram p7: hidden frame]
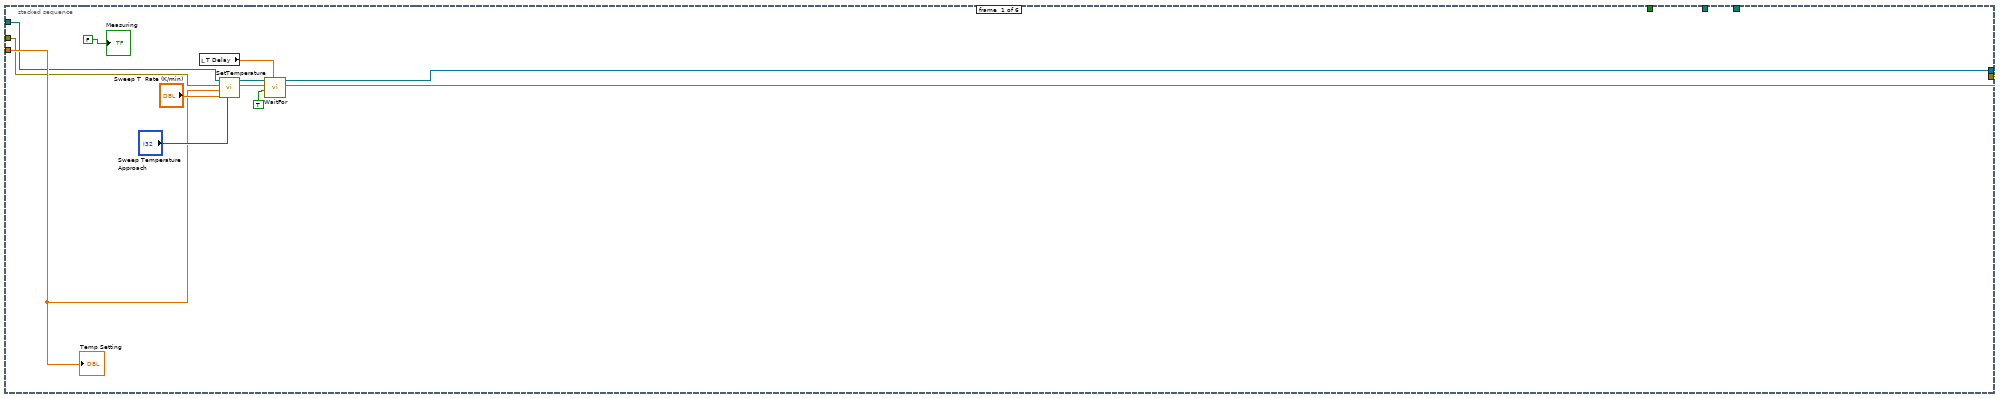
[diagram p8: hidden frame]
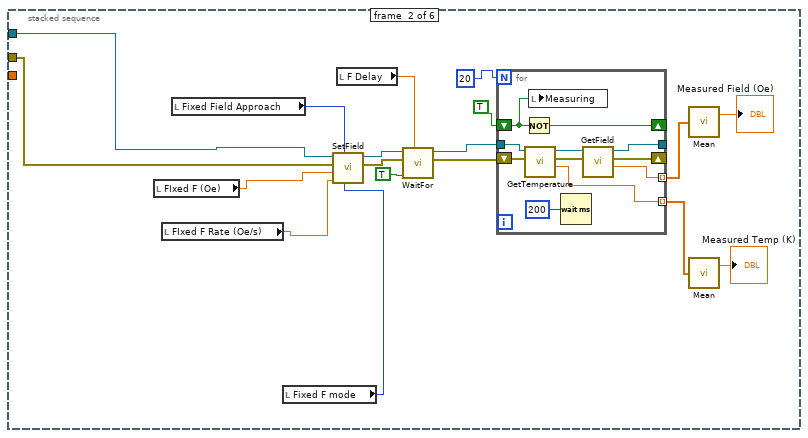
[diagram p9: hidden frame]
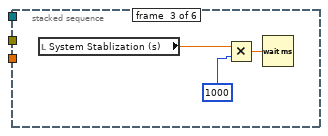
[diagram p10: hidden frame]
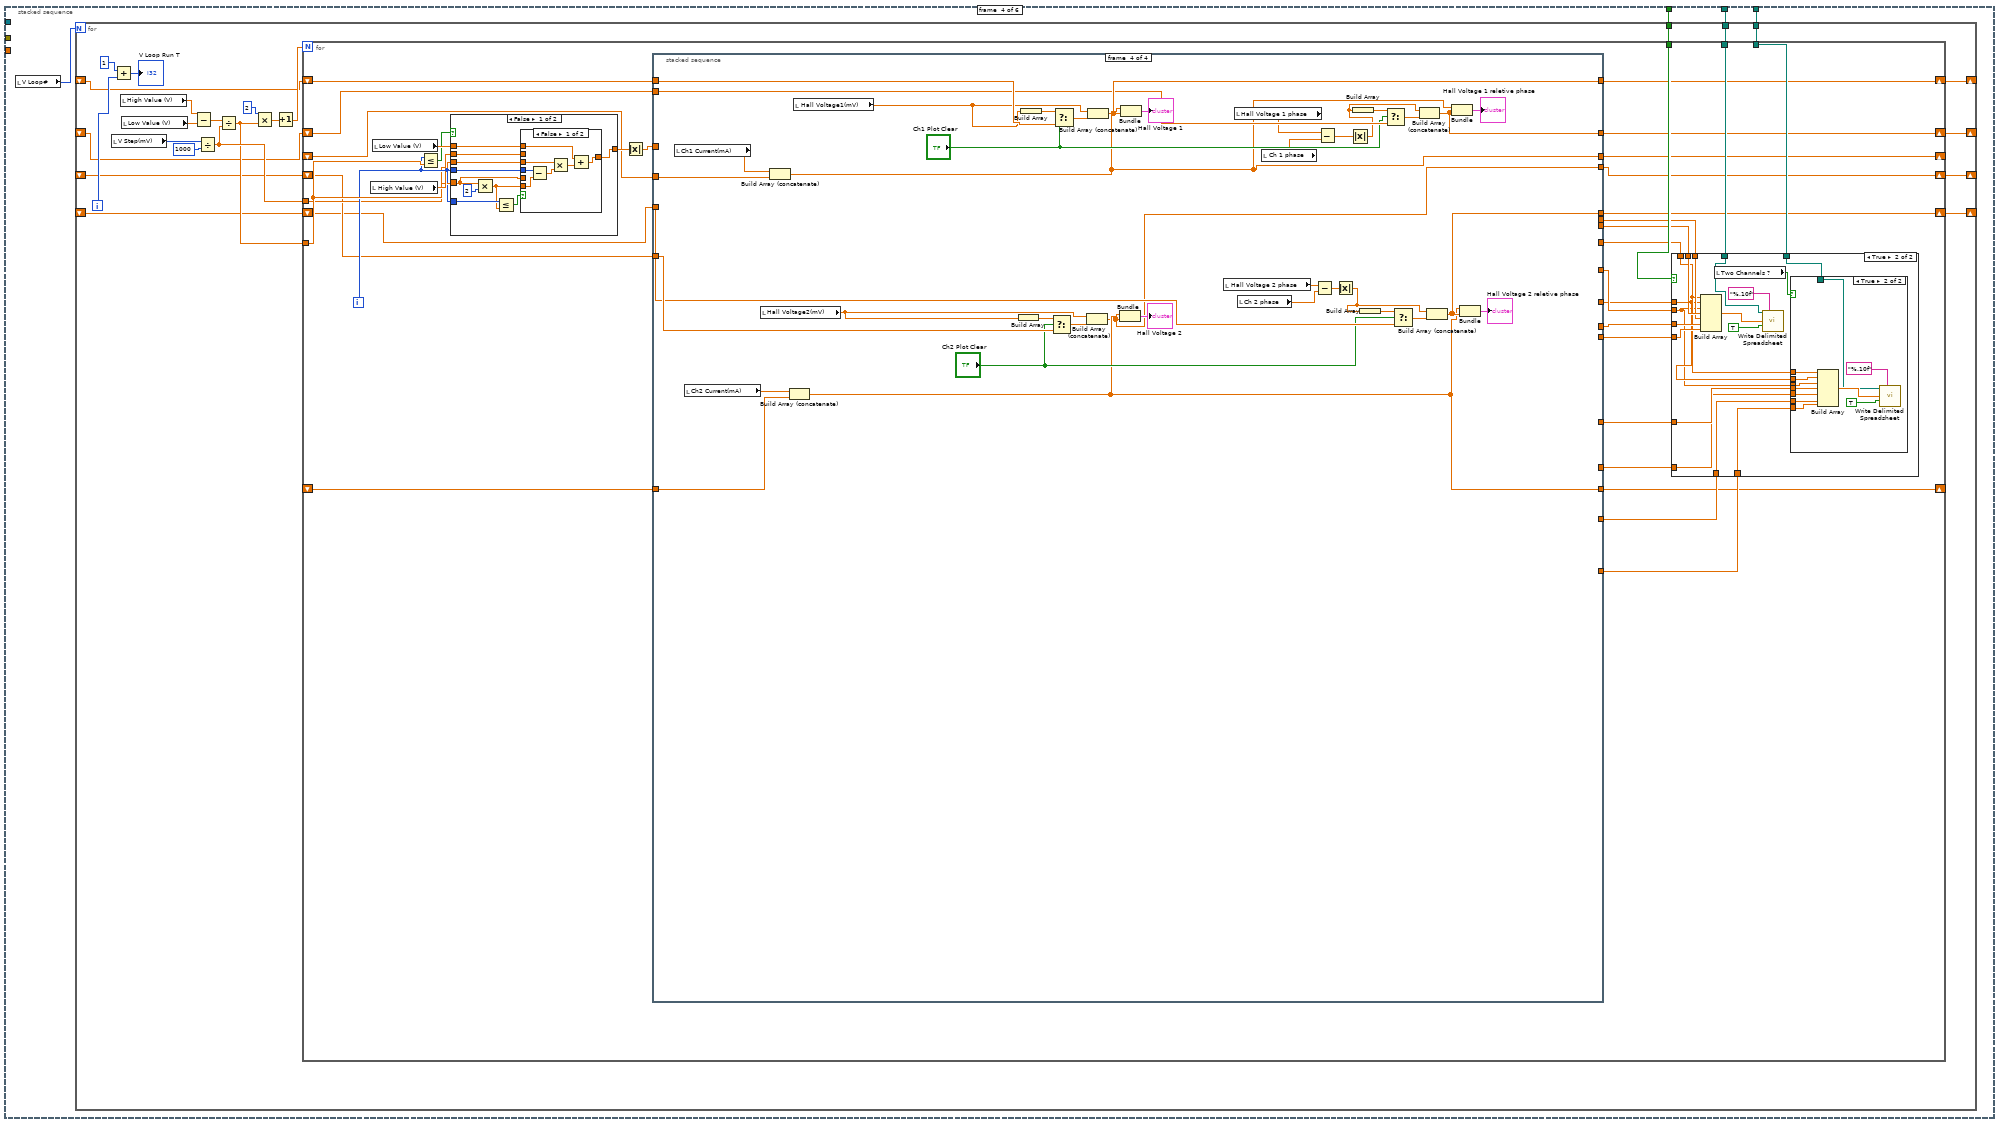
[diagram p11: hidden frame]
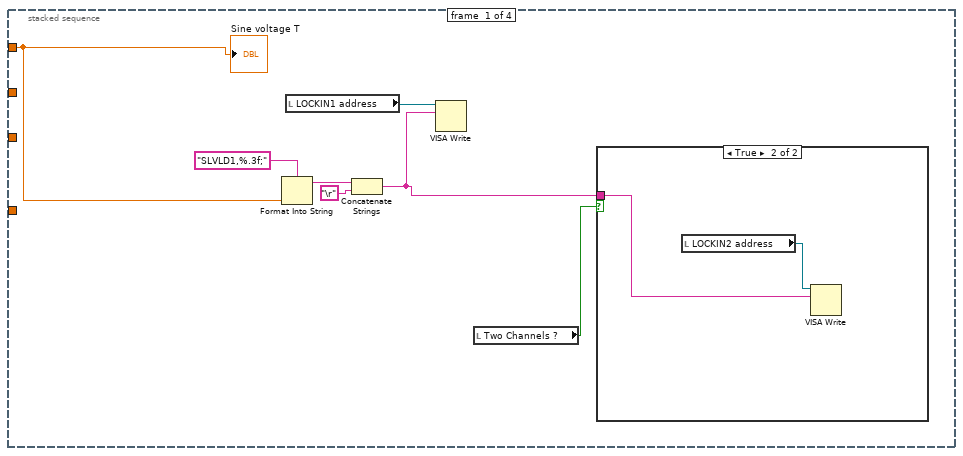
[diagram p12: hidden frame]
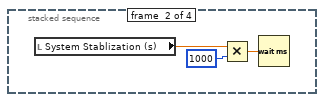
[diagram p14: hidden frame]
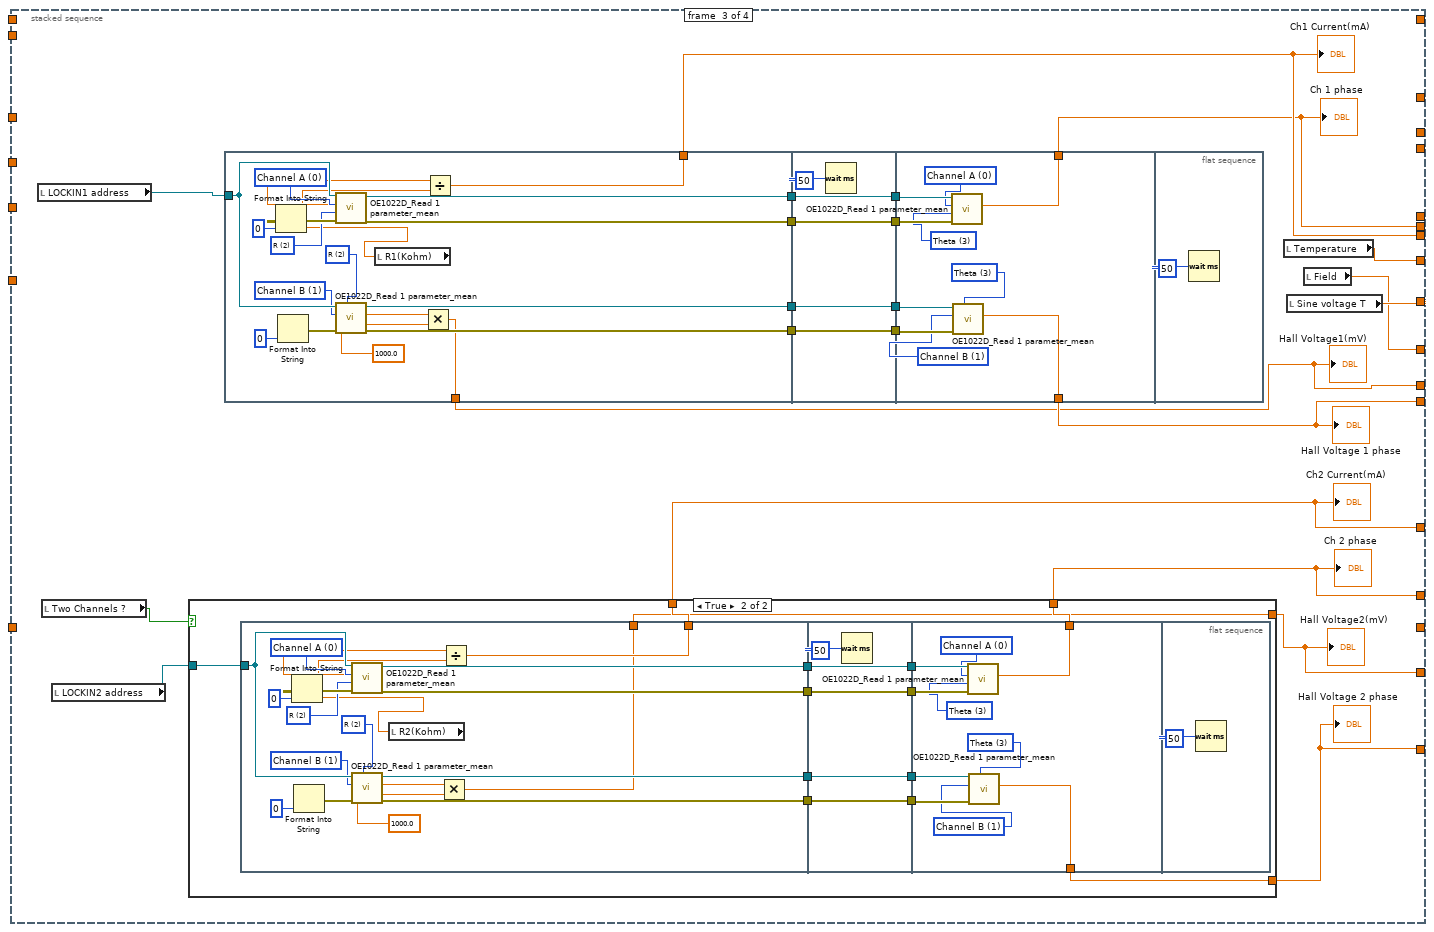
[diagram p15: hidden frame]
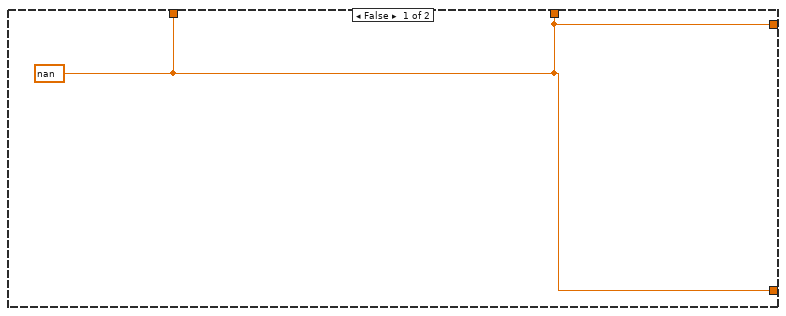
[diagram p16: hidden frame]
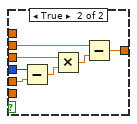
[diagram p17: hidden frame]
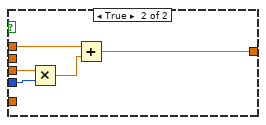
[diagram p18: hidden frame]
diagram:
  w23 = "Sweep T"
  w18 = ".txt"
  n1 = flat-sequence {
    tunnel: [w38] -> w36
    tunnel: [w37] -> w35
    tunnel: [w38] -> w32
    tunnel: [w37] -> w31
    tunnel: w36 -> [w51]
    tunnel: w35 -> [w50]
    tunnel: [w49] -> w34
    tunnel: [w48] -> w33
    tunnel: w17 -> [w44]
    tunnel: w16 -> [w43]
    tunnel: "Save data or not" -> [w42]
    tunnel: w34 -> [w935]
    tunnel: w33 -> [w934]
    frame #0 {
      w39 = 4 items=["PPMS", "VersaLab", "DynaCool", "SVSM", "OptiCool"] ("InstrumentType")
      n2 = call "OpenQDInstrument.vi"("Remote"="Remote", "IP Address"="IP Address", "InstrumentType"=w39) -> ("error out"=w37:errorcluster, "Instrument Ref"=w38:refnum<k24>)  [unwired: 5 in]
    }
    frame #1 {
      n3 = case shown="True" "Two Channels ?" {
        frame False {
        }
        frame True {
        }
      }
      n4 = stacked-sequence {
        tunnel: "Single/Double" -> [_ w261]
        tunnel: w51 -> [_ w245]
        tunnel: w50 -> [_ w246]
        tunnel: [_ w260] -> w49
        tunnel: [_ w259] -> w48
        tunnel: w44 -> [_ w257]
        tunnel: w43 -> [_ w256]
        tunnel: w42 -> [_ w258]
        frame #0 {
          n5 = local read "Two Channels ?"() -> (w53:bool)
          n6 = local read "LOCKIN1 address"() -> (w54:refnum<visa-resource-name>)
          n7 = call "OE1022D_OpenDevice.vi"("VISA resource name"=w54) -> ("VISA资源名称输出"=w55:refnum<visa-resource-name>, "错误输出"=w56:errorcluster)  [unwired: 17 in]
          n8 = call "OE1022D_Abort.vi"("error in (no error)"=w56, "VISA resource name"=w55) -> ("error out"=w61:errorcluster, "VISA resource name out"=w62:refnum<visa-resource-name>)
          n9 = case shown="True" w53 {
            frame False {
            }
            frame True {
              n10 = local read "LOCKIN2 address"() -> (w64:refnum<visa-resource-name>)
              n11 = call "OE1022D_OpenDevice.vi"("VISA resource name"=w64) -> ("VISA资源名称输出"=w67:refnum<visa-resource-name>, "错误输出"=w68:errorcluster)  [unwired: 17 in]
              n12 = call "OE1022D_Abort.vi"("error in (no error)"=w68, "VISA resource name"=w67) -> ("error out"=w65:errorcluster, "VISA resource name out"=w66:refnum<visa-resource-name>)
              n13 = flat-sequence {
                tunnel: w66 -> [w113]
                tunnel: [w101] -> w73
                tunnel: w65 -> [w112]
                tunnel: [w89] -> w72
                tunnel: w73 -> [w118]
                tunnel: [w118] -> w71
                tunnel: w72 -> [w117]
                tunnel: [w117] -> w70
                tunnel: w71 -> [w140]
                tunnel: [w139] -> w69
                tunnel: w70 -> [w138]
                tunnel: w69 -> [_]
                frame #0 {
                  w74 = u8 2 items=["TTL Pos", "TTL Neg", "Sine Zero Crossing"] ("External Ref Trigger")
                  w75 = u8 1 items=["Single", "Loop"] ("Sample Mode (Single/Loop)")
                  w88 = u8 0 items=["Fixed", "Linear", "Log"] ("SineOut Mode")
                  w90 = u16 0 items=["Internal", "External"] ("Trigger Source (0: Internal)")
                  w79 = u8 0 items=["Channel A", "Channel B"] ("OE1022D A/B")
                  n14 = call "OE1022D_Configure Trigger.vi"("Trigger Source (0: Internal)"=w90, "error in (no error)   2"=w112, "OE1022D A/B"=w79, "VISA resource name   2"=w113) -> ("error out   2"=w106:errorcluster, "VISA resource name out   2"=w107:refnum<visa-resource-name>)
                  n15 = call "OE1022D_Configure Reference Source.vi"("VISA resource name"=w107, "OE1022D A/B"=w79, "Reference Source"="2A Reference Source", "error in (no error)"=w106) -> ("VISA resource name out"=w105:refnum<visa-resource-name>, "error out"=w103:errorcluster)  [unwired: 14 in]
                  n16 = call "OE1022D_Configure Harmonic.vi"("VISA resource name"=w105, "OE1022D A/B"=w79, "Harmonic 1"="2A harmonic 1", "Harmonic 2"="2A harmonic 2", "error in (no error)"=w103) -> ("VISA resource name out"=w104:refnum<visa-resource-name>, "error out"=w102:errorcluster)  [unwired: 13 in]
                  n17 = call "OE1022D_Configure Sine Out.vi"("VISA resource name"=w104, "SineOut Mode"=w88, "OE1022D A/B"=w79, "Sine Output Amplitude (V)"=sgl 0.001, "error in (no error)"=w102) -> ("VISA resource name out"=w110:refnum<visa-resource-name>, "error out"=w109:errorcluster)  [unwired: 9 in]
                  n18 = call "OE1022D_Configure Frequency.vi"("VISA resource name"=w110, "OE1022D A/B"=w79, "Internal Frequency(Hz)"="2A frequency", "error in (no error)"=w109) -> ("VISA resource name out"=w100:refnum<visa-resource-name>, "error out"=w97:errorcluster)  [unwired: 14 in]
                  n19 = call "OE1022D_Configure Ref Phase Channel A.vi"("VISA resource name"=w100, "Reference Source"="2A Reference Source", "External Ref Trigger"=w74, "Internal Frequency(Hz)"="2A frequency", "Auto Phase (T: Enabled)"="auto phase 2A", "error in (no error)"=w97, "Manual Phase  (degree)"="2A reference Manual Phase") -> ("VISA resource name out"=w99:refnum<visa-resource-name>, "error out"=w98:errorcluster)  [unwired: 11 in]
                  n20 = call "OE1022D_Configure_Acquisition.vi"("VISA resource name"=w99, "OE1022D A/B"=w79, "Sample time (s)"="2A Sample time (s)", "error in (no error)"=w98, "Sample Mode (Single/Loop)"=w75) -> ("VISA resource name out"=w82:refnum<visa-resource-name>, "error out"=w81:errorcluster)  [unwired: 3 in]
                  n21 = call "OE1022D_Configure Sensitivity.vi"("VISA resource name"=w82, "OE1022D A/B"=w79, "Sensitivity"="2A Sensitivity", "error in (no error)"=w81) -> ("VISA resource name out"=w86:refnum<visa-resource-name>, "error out"=w85:errorcluster)  [unwired: 14 in]
                  n22 = call "OE1022D_Configure Filter.vi"("Low Pass Filter Slope (1: 12dB/oct)"="2A Low Pass Filter Slope", "Time Constant (8: 100ms)"="2A Time Constant", "error in (no error)"=w85, "Enable Sync Filter (F: Disable)"="Enable Sync Filter 2A (open when f<200Hz)", "OE1022D A/B"=w79, "VISA resource name"=w86) -> ("error out"=w83:errorcluster, "VISA resource name out"=w84:refnum<visa-resource-name>)  [unwired: 4 in]
                  n23 = call "OE1022D_Configure Input Filter.vi"("VISA resource name"=w84, "Input Source"="2A Input Connection (0: Single-Ended)", "OE1022D A/B"=w79, "error in (no error)"=w83) -> ("VISA resource name out"=w89:refnum<visa-resource-name>, "error out"=w101:errorcluster)  [unwired: 10 in]
                }
                frame #1 {
                  n24 = local read "System Stablization (s)"() -> (w114:dbl)
                  n25 = Multiply(x=w114, y=1000) -> (x*y=w116:dbl)
                  n26 = Wait (ms)(milliseconds to wait=w116) -> ()  [unwired: 1 out]
                }
                frame #2 {
                  w120 = u8 1 items=["Single", "Loop"] ("Sample Mode (Single/Loop)")
                  w122 = u8 2 items=["TTL Pos", "TTL Neg", "Sine Zero Crossing"] ("External Ref Trigger")
                  w135 = u8 0 items=["Fixed", "Linear", "Log"] ("SineOut Mode")
                  w141 = u16 0 items=["Internal", "External"] ("Trigger Source (0: Internal)")
                  w127 = u8 1 items=["Channel A", "Channel B"] ("OE1022D A/B")
                  n27 = call "OE1022D_Configure Trigger.vi"("Trigger Source (0: Internal)"=w141, "error in (no error)   2"=w140, "OE1022D A/B"=w127, "VISA resource name   2"=w138) -> ("error out   2"=w153:errorcluster, "VISA resource name out   2"=w154:refnum<visa-resource-name>)
                  n28 = call "OE1022D_Configure Reference Source.vi"("VISA resource name"=w154, "OE1022D A/B"=w127, "error in (no error)"=w153) -> ("VISA resource name out"=w152:refnum<visa-resource-name>, "error out"=w150:errorcluster)  [unwired: 15 in]
                  n29 = call "OE1022D_Configure Harmonic.vi"("VISA resource name"=w152, "OE1022D A/B"=w127, "Harmonic 1"="2B harmonic 1", "Harmonic 2"="2B harmonic 2", "error in (no error)"=w150) -> ("VISA resource name out"=w151:refnum<visa-resource-name>, "error out"=w149:errorcluster)  [unwired: 13 in]
                  n30 = call "OE1022D_Configure Sine Out.vi"("VISA resource name"=w151, "SineOut Mode"=w135, "OE1022D A/B"=w127, "Sine Output Amplitude (V)"=sgl 0.001, "error in (no error)"=w149) -> ("VISA resource name out"=w156:refnum<visa-resource-name>, "error out"=w155:errorcluster)  [unwired: 9 in]
                  n31 = call "OE1022D_Configure Frequency.vi"("VISA resource name"=w156, "OE1022D A/B"=w127, "Internal Frequency(Hz)"="2B frequency 2", "error in (no error)"=w155) -> ("VISA resource name out"=w148:refnum<visa-resource-name>, "error out"=w145:errorcluster)  [unwired: 14 in]
                  n32 = call "OE1022D_Configure Ref Phase Channel B.vi"("VISA resource name"=w148, "Reference Source"="2B Reference Source", "External Ref Trigger"=w122, "Internal Frequency(Hz)"="2B frequency 2", "Auto Phase (T: Enabled)"="auto phase 2B", "error in (no error)"=w145, "Manual Phase  (degree)"="2B reference Manual Phase") -> ("VISA resource name out"=w147:refnum<visa-resource-name>, "error out"=w146:errorcluster)  [unwired: 11 in]
                  n33 = call "OE1022D_Configure_Acquisition.vi"("VISA resource name"=w147, "OE1022D A/B"=w127, "Sample time (s)"="2B Sample time (s)", "error in (no error)"=w146, "Sample Mode (Single/Loop)"=w120) -> ("VISA resource name out"=w128:refnum<visa-resource-name>, "error out"=w129:errorcluster)  [unwired: 3 in]
                  n34 = call "OE1022D_Configure Sensitivity.vi"("VISA resource name"=w128, "OE1022D A/B"=w127, "Sensitivity"="2B Sensitivity", "error in (no error)"=w129) -> ("VISA resource name out"=w132:refnum<visa-resource-name>, "error out"=w131:errorcluster)  [unwired: 14 in]
                  n35 = call "OE1022D_Configure Filter.vi"("Low Pass Filter Slope (1: 12dB/oct)"="2B Low Pass Filter Slope", "Time Constant (8: 100ms)"="2B Time Constant", "error in (no error)"=w131, "Enable Sync Filter (F: Disable)"="Enable Sync Filter 2B (open when f<200Hz)", "OE1022D A/B"=w127, "VISA resource name"=w132) -> ("error out"=w130:errorcluster, "VISA resource name out"=w119:refnum<visa-resource-name>)  [unwired: 4 in]
                  n36 = call "OE1022D_Configure Input Filter.vi"("VISA resource name"=w119, "Input Source"="2B Input Connection (0: Single-Ended)", "OE1022D A/B"=w127, "error in (no error)"=w130) -> ("error out"=w139:errorcluster)  [unwired: 10 in, 1 out]
                }
                frame #3 {
                  n37 = local read "System Stablization (s)"() -> (w158:dbl)
                  n38 = Multiply(x=w158, y=1000) -> (x*y=w160:dbl)
                  n39 = Wait (ms)(milliseconds to wait=w160) -> ()  [unwired: 1 out]
                }
              }
            }
          }
          n40 = flat-sequence {
            tunnel: w62 -> [w198]
            tunnel: [w186] -> w60
            tunnel: w61 -> [w197]
            tunnel: [w174] -> w58
            tunnel: w60 -> [w203]
            tunnel: [w203] -> w59
            tunnel: w58 -> [w202]
            tunnel: [w202] -> w57
            tunnel: w59 -> [w224]
            tunnel: [w223] -> w63
            tunnel: w57 -> [w222]
            tunnel: w63 -> [_]
            frame #0 {
              w173 = u8 0 items=["Fixed", "Linear", "Log"] ("SineOut Mode")
              w175 = u16 0 items=["Internal", "External"] ("Trigger Source (0: Internal)")
              w164 = u8 0 items=["Channel A", "Channel B"] ("OE1022D A/B")
              n41 = call "OE1022D_Configure Trigger.vi"("Trigger Source (0: Internal)"=w175, "error in (no error)   2"=w197, "OE1022D A/B"=w164, "VISA resource name   2"=w198) -> ("error out   2"=w191:errorcluster, "VISA resource name out   2"=w192:refnum<visa-resource-name>)
              n42 = call "OE1022D_Configure Reference Source.vi"("VISA resource name"=w192, "OE1022D A/B"=w164, "Reference Source"="A Reference Source", "error in (no error)"=w191) -> ("VISA resource name out"=w190:refnum<visa-resource-name>, "error out"=w188:errorcluster)  [unwired: 14 in]
              n43 = call "OE1022D_Configure Harmonic.vi"("VISA resource name"=w190, "OE1022D A/B"=w164, "Harmonic 1"="A harmonic 1", "Harmonic 2"="A harmonic 2", "error in (no error)"=w188) -> ("VISA resource name out"=w189:refnum<visa-resource-name>, "error out"=w187:errorcluster)  [unwired: 13 in]
              n44 = call "OE1022D_Configure Sine Out.vi"("VISA resource name"=w189, "SineOut Mode"=w173, "OE1022D A/B"=w164, "Sine Output Amplitude (V)"=sgl 0.001 ("A Sine Output Amplitude (V)"), "error in (no error)"=w187) -> ("VISA resource name out"=w195:refnum<visa-resource-name>, "error out"=w194:errorcluster)  [unwired: 9 in]
              n45 = call "OE1022D_Configure Frequency.vi"("VISA resource name"=w195, "OE1022D A/B"=w164, "Internal Frequency(Hz)"="A frequency", "error in (no error)"=w194) -> ("VISA resource name out"=w185:refnum<visa-resource-name>, "error out"=w182:errorcluster)  [unwired: 14 in]
              n46 = call "OE1022D_Configure Ref Phase Channel A.vi"("VISA resource name"=w185, "Reference Source"="A Reference Source", "Internal Frequency(Hz)"="A frequency", "Auto Phase (T: Enabled)"="auto phase A", "error in (no error)"=w182, "Manual Phase  (degree)"="A reference Manual Phase") -> ("VISA resource name out"=w184:refnum<visa-resource-name>, "error out"=w183:errorcluster)  [unwired: 12 in]
              n47 = call "OE1022D_Configure_Acquisition.vi"("VISA resource name"=w184, "OE1022D A/B"=w164, "Sample time (s)"="A Sample time (s)", "error in (no error)"=w183) -> ("VISA resource name out"=w167:refnum<visa-resource-name>, "error out"=w166:errorcluster)  [unwired: 4 in]
              n48 = call "OE1022D_Configure Sensitivity.vi"("VISA resource name"=w167, "OE1022D A/B"=w164, "Sensitivity"="A Sensitivity", "error in (no error)"=w166) -> ("VISA resource name out"=w171:refnum<visa-resource-name>, "error out"=w170:errorcluster)  [unwired: 14 in]
              n49 = call "OE1022D_Configure Filter.vi"("Low Pass Filter Slope (1: 12dB/oct)"="A Low Pass Filter Slope", "Time Constant (8: 100ms)"="A Time Constant", "error in (no error)"=w170, "Enable Sync Filter (F: Disable)"="Enable Sync Filter A (open when f<200Hz)", "OE1022D A/B"=w164, "VISA resource name"=w171) -> ("error out"=w168:errorcluster, "VISA resource name out"=w169:refnum<visa-resource-name>)  [unwired: 4 in]
              n50 = call "OE1022D_Configure Input Filter.vi"("VISA resource name"=w169, "Input Source"="A Input Connection (0: Single-Ended)", "OE1022D A/B"=w164, "error in (no error)"=w168) -> ("VISA resource name out"=w174:refnum<visa-resource-name>, "error out"=w186:errorcluster)  [unwired: 10 in]
            }
            frame #1 {
              n51 = local read "System Stablization (s)"() -> (w199:dbl)
              n52 = Multiply(x=w199, y=1000) -> (x*y=w201:dbl)
              n53 = Wait (ms)(milliseconds to wait=w201) -> ()  [unwired: 1 out]
            }
            frame #2 {
              w206 = u8 2 items=["TTL Pos", "TTL Neg", "Sine Zero Crossing"] ("External Ref Trigger")
              w219 = u8 0 items=["Fixed", "Linear", "Log"] ("SineOut Mode")
              w225 = u16 0 items=["Internal", "External"] ("Trigger Source (0: Internal)")
              w211 = u8 1 items=["Channel A", "Channel B"] ("OE1022D A/B")
              n54 = call "OE1022D_Configure Trigger.vi"("Trigger Source (0: Internal)"=w225, "error in (no error)   2"=w224, "OE1022D A/B"=w211, "VISA resource name   2"=w222) -> ("error out   2"=w237:errorcluster, "VISA resource name out   2"=w238:refnum<visa-resource-name>)
              n55 = call "OE1022D_Configure Reference Source.vi"("VISA resource name"=w238, "OE1022D A/B"=w211, "error in (no error)"=w237) -> ("VISA resource name out"=w236:refnum<visa-resource-name>, "error out"=w234:errorcluster)  [unwired: 15 in]
              n56 = call "OE1022D_Configure Harmonic.vi"("VISA resource name"=w236, "OE1022D A/B"=w211, "Harmonic 1"="B harmonic 1", "Harmonic 2"="B harmonic 2", "error in (no error)"=w234) -> ("VISA resource name out"=w235:refnum<visa-resource-name>, "error out"=w233:errorcluster)  [unwired: 13 in]
              n57 = call "OE1022D_Configure Sine Out.vi"("VISA resource name"=w235, "SineOut Mode"=w219, "OE1022D A/B"=w211, "Sine Output Amplitude (V)"=sgl 0.001, "error in (no error)"=w233) -> ("VISA resource name out"=w240:refnum<visa-resource-name>, "error out"=w239:errorcluster)  [unwired: 9 in]
              n58 = call "OE1022D_Configure Frequency.vi"("VISA resource name"=w240, "OE1022D A/B"=w211, "Internal Frequency(Hz)"="B frequency", "error in (no error)"=w239) -> ("VISA resource name out"=w232:refnum<visa-resource-name>, "error out"=w229:errorcluster)  [unwired: 14 in]
              n59 = call "OE1022D_Configure Ref Phase Channel B.vi"("VISA resource name"=w232, "Reference Source"="B Reference Source", "External Ref Trigger"=w206, "Internal Frequency(Hz)"="B frequency", "Auto Phase (T: Enabled)"="auto phase B", "error in (no error)"=w229, "Manual Phase  (degree)"="B reference Manual Phase") -> ("VISA resource name out"=w231:refnum<visa-resource-name>, "error out"=w230:errorcluster)  [unwired: 11 in]
              n60 = call "OE1022D_Configure_Acquisition.vi"("VISA resource name"=w231, "OE1022D A/B"=w211, "Sample time (s)"="B Sample time (s)", "error in (no error)"=w230) -> ("VISA resource name out"=w212:refnum<visa-resource-name>, "error out"=w213:errorcluster)  [unwired: 4 in]
              n61 = call "OE1022D_Configure Sensitivity.vi"("VISA resource name"=w212, "OE1022D A/B"=w211, "Sensitivity"="B Sensitivity", "error in (no error)"=w213) -> ("VISA resource name out"=w216:refnum<visa-resource-name>, "error out"=w215:errorcluster)  [unwired: 14 in]
              n62 = call "OE1022D_Configure Filter.vi"("Low Pass Filter Slope (1: 12dB/oct)"="B Low Pass Filter Slope", "Time Constant (8: 100ms)"="B Time Constant", "error in (no error)"=w215, "Enable Sync Filter (F: Disable)"="Enable Sync Filter B (open when f<200Hz)", "OE1022D A/B"=w211, "VISA resource name"=w216) -> ("error out"=w214:errorcluster, "VISA resource name out"=w204:refnum<visa-resource-name>)  [unwired: 4 in]
              n63 = call "OE1022D_Configure Input Filter.vi"("VISA resource name"=w204, "Input Source"="B Input Connection (0: Single-Ended)", "OE1022D A/B"=w211, "error in (no error)"=w214) -> ("error out"=w223:errorcluster)  [unwired: 10 in, 1 out]
            }
            frame #3 {
              n64 = local read "System Stablization (s)"() -> (w242:dbl)
              n65 = Multiply(x=w242, y=1000) -> (x*y=w244:dbl)
              n66 = Wait (ms)(milliseconds to wait=w244) -> ()  [unwired: 1 out]
            }
          }
        }
        frame #1 {
          n67 = Subtract(x="End Value (K)", y="Start Value (K)") -> (x-y=w253:dbl)
          n68 = Divide(x="Step(K)", y=1) -> (x/y=w252:dbl)
          n69 = Divide(x=w253, y=w252) -> (x/y=w251:dbl)
          n70 = Multiply(x=w261, y=w251) -> (x*y=w250:dbl)
          n71 = Increment(x=w250) -> (x+1=w249:dbl)
          n72 = for {
            N: w249 -> [_]
            tunnel: w252 -> [w274]
            tunnel: w251 -> [w272]
            tunnel: "Start Value (K)" -> [w275]
            tunnel: "End Value (K)" -> [w273]
            tunnel: w245 -> [w268]
            tunnel: w246 -> [w267]
            tunnel: [w266] -> w260
            tunnel: [w262] -> w259
            tunnel: w258 -> [w265]
            tunnel: w257 -> [w264]
            tunnel: w256 -> [w263]
            i -> [w271]
            n73 = Less Or Equal?(x=w271, y=w272) -> (x <= y?=w276:bool)
            n74 = case shown="False" w276 {
              selector: w276 -> [w277 w303]
              tunnel: w275 -> [w279 w308]
              tunnel: w271 -> [w288 w307]
              tunnel: w274 -> [w287 w306]
              tunnel: [w285 w304] -> w270
              tunnel: w273 -> [w286 _]
              tunnel: w272 -> [w281 _]
              tunnel: w271 -> [w284 _]
              frame False {
                n75 = local write "Forward"(w277) -> ()
                n76 = Not(x=w277) -> (.not. x?=w278:bool)
                n77 = Multiply(x=w281, y=2) -> (x*y=w280:dbl)
                n78 = Less Or Equal?(x=w284, y=w280) -> (x <= y?=w282:bool)
                n79 = local write "Backward"(w278) -> ()
                n80 = case shown="True" w282 {
                  tunnel: w288 -> [w295 w302]
                  tunnel: w287 -> [w293 w300]
                  tunnel: w286 -> [_ w298]
                  tunnel: [w291 w297] -> w285
                  tunnel: w281 -> [_ w296]
                  tunnel: w280 -> [w290 _]
                  tunnel: w279 -> [w289 _]
                  frame False {
                    n81 = Subtract(x=w295, y=w290) -> (x-y=w294:dbl)
                    n82 = Multiply(x=w293, y=w294) -> (x*y=w292:dbl)
                    n83 = Add(x=w289, y=w292) -> (x+y=w291:dbl)
                  }
                  frame True {
                    n84 = Subtract(x=w302, y=w296) -> (x-y=w301:dbl)
                    n85 = Multiply(x=w300, y=w301) -> (x*y=w299:dbl)
                    n86 = Subtract(x=w298, y=w299) -> (x-y=w297:dbl)
                  }
                }
              }
              frame True {
                n87 = Multiply(x=w306, y=w307) -> (x*y=w305:dbl)
                n88 = local write "Forward"(w303) -> ()
                n89 = Add(x=w308, y=w305) -> (x+y=w304:dbl)
              }
            }
            n90 = Absolute Value(x=w270) -> (abs(x)=w269:dbl)
            n91 = stacked-sequence {
              tunnel: w269 -> [w317 _ _ _ _ _]
              tunnel: w268 -> [w316 w334 _ _ w629 _]
              tunnel: w267 -> [w315 w335 _ _ w628 _]
              tunnel: [w309 _ _ _ _ _] -> w266
              tunnel: [w310 _ _ _ _ _] -> w262
              tunnel: w265 -> [_ _ _ w355 _ w660]
              tunnel: w264 -> [_ _ _ w354 _ w659]
              tunnel: w263 -> [_ _ _ w353 _ w658]
              frame #0 {
                n92 = local read "T Delay"() -> (w311:dbl)
                n93 = call "SetTemperature.vi"("Approach"="Sweep Temperature Approach", "Rate"="Sweep T  Rate (K/min)", "Temperature"=w317, "error in (no error)"=w315, "Instrument Ref In"=w316) -> ("error out"=w313:errorcluster, "Instrument Ref Out"=w314:refnum<k24>)  [unwired: 2 in, 1 out]
                n94 = call "WaitFor.vi"("Delay"=w311, "Wait For Temperature"=TRUE ("WaitForTemperature"), "error in (no error)"=w313, "Instrument Ref In"=w314) -> ("error out"=w309:errorcluster, "Instrument Ref Out"=w310:refnum<k24>)  [unwired: 6 in]
                "Temp Setting" <- w317
                "Measuring" <- FALSE
              }
              frame #1 {
                n95 = local read "FIxed F (Oe)"() -> (w330:dbl)
                n96 = local read "FIxed F Rate (Oe/s)"() -> (w331:dbl)
                n97 = local read "Fixed Field Approach"() -> (w329:i32)
                n98 = local read "Fixed F mode"() -> (w332:i32)
                n99 = call "SetField.vi"("Mode"=w332, "Approach"=w329, "Rate"=w331, "Field"=w330, "error in (no error)"=w335, "Instrument Ref In"=w334) -> ("error out"=w337:errorcluster, "Instrument Ref Out"=w338:refnum<k24>)  [unwired: 1 in, 1 out]
                n100 = local read "F Delay"() -> (w333:dbl)
                n101 = call "WaitFor.vi"("Delay"=w333, "Wait For Field"=TRUE, "error in (no error)"=w337, "Instrument Ref In"=w338) -> ("error out"=w321:errorcluster, "Instrument Ref Out"=w322:refnum<k24>)  [unwired: 6 in]
                n102 = for {
                  N: 20 -> [_]
                  shift-right: [w349] -> _
                  shift-left: TRUE -> [w347]
                  shift-right: [w344] -> _
                  shift-left: w321 -> [w346]
                  tunnel: w322 -> [w343]
                  tunnel: [w341] -> _
                  tunnel: [w339] -> w325 mode=indexing
                  tunnel: [w340] -> w326 mode=indexing
                  n103 = Not(x=w347) -> (.not. x?=w349:bool)
                  n104 = call "GetTemperature.vi"("error in (no error)"=w346, "Instrument Ref In"=w343) -> ("Temperature"=w340:dbl, "error out"=w345:errorcluster, "Instrument Ref Out"=w342:refnum<k24>)  [unwired: 3 in, 2 out]
                  n105 = local write "Measuring"(w347) -> ()
                  n106 = Wait (ms)(milliseconds to wait=u32 200) -> ()  [unwired: 1 out]
                  n107 = call "GetField.vi"("error in (no error)"=w345, "Instrument Ref In"=w342) -> ("Field"=w339:dbl, "error out"=w344:errorcluster, "Instrument Ref Out"=w341:refnum<k24>)  [unwired: 3 in, 2 out]
                }
                n108 = call-poly <vilib>:"Mean.vi"("X"=w325) -> ("mean"=→"Measured Field (Oe)":dbl)  [unwired: 1 out]
                n109 = call-poly <vilib>:"Mean.vi"("X"=w326) -> ("mean"=→"Measured Temp (K)":dbl)  [unwired: 1 out]
              }
              frame #2 {
                n110 = local read "System Stablization (s)"() -> (w350:dbl)
                n111 = Multiply(x=w350, y=1000) -> (x*y=w352:dbl)
                n112 = Wait (ms)(milliseconds to wait=w352) -> ()  [unwired: 1 out]
              }
              frame #3 {
                n113 = local read "V Loop#"() -> (w356:i32)
                n114 = for {
                  N: w356 -> [_]
                  tunnel: w355 -> [w367]
                  tunnel: w354 -> [w366]
                  tunnel: w353 -> [w365]
                  shift-right: [w364] -> _
                  shift-left: _ -> [w363]
                  shift-right: [w362] -> _
                  shift-left: _ -> [w361]
                  shift-right: [w360] -> _
                  shift-left: _ -> [w359]
                  shift-right: [w358] -> _
                  shift-left: _ -> [w357]
                  i -> [w380]
                  n115 = local read "V Step(mV)"() -> (w368:i32)
                  n116 = Add(x=1, y=w380) -> (x+y=→"V Loop Run T":i32)
                  n117 = local read "High Value (V)"() -> (w370:dbl)
                  n118 = local read "Low Value (V)"() -> (w369:dbl)
                  n119 = Subtract(x=w370, y=w369) -> (x-y=w375:dbl)
                  n120 = Divide(x=w368, y=1000) -> (x/y=w372:dbl)
                  n121 = Divide(x=w375, y=w372) -> (x/y=w371:dbl)
                  n122 = Multiply(x=2, y=w371) -> (x*y=w374:dbl)
                  n123 = Increment(x=w374) -> (x+1=w373:dbl)
                  n124 = for {
                    N: w373 -> [_]
                    tunnel: w372 -> [w409]
                    tunnel: w371 -> [w411]
                    tunnel: w367 -> [w406]
                    tunnel: w366 -> [w405]
                    tunnel: w365 -> [w404]
                    shift-right: [w402] -> w364
                    shift-left: w363 -> [w401]
                    shift-right: [w400] -> w362
                    shift-left: w361 -> [w399]
                    shift-right: [w398] -> w360
                    shift-left: w359 -> [w397]
                    shift-right: [w396] -> w358
                    shift-left: w357 -> [w395]
                    shift-right: [w384] -> _
                    shift-left: _ -> [w383]
                    shift-right: [w382] -> _
                    shift-left: _ -> [w381]
                    i -> [w410]
                    n125 = local read "High Value (V)"() -> (w413:dbl)
                    n126 = local read "Low Value (V)"() -> (w414:dbl)
                    n127 = Less Or Equal?(x=w410, y=w411) -> (x <= y?=w412:bool)
                    n128 = case shown="False" w412 {
                      tunnel: w414 -> [w571 w599]
                      tunnel: w410 -> [w580 w598]
                      tunnel: w409 -> [w579 w597]
                      tunnel: [w577 w595] -> w408
                      tunnel: w413 -> [w578 _]
                      tunnel: w411 -> [w573 _]
                      tunnel: w410 -> [w576 _]
                      frame False {
                        n129 = Multiply(x=w573, y=2) -> (x*y=w572:dbl)
                        n130 = Less Or Equal?(x=w576, y=w572) -> (x <= y?=w574:bool)
                        n131 = case shown="False" w574 {
                          tunnel: w580 -> [w587 w594]
                          tunnel: w579 -> [w585 w592]
                          tunnel: w578 -> [_ w590]
                          tunnel: [w583 w589] -> w577
                          tunnel: w573 -> [_ w588]
                          tunnel: w572 -> [w582 _]
                          tunnel: w571 -> [w581 _]
                          frame False {
                            n132 = Subtract(x=w587, y=w582) -> (x-y=w586:dbl)
                            n133 = Multiply(x=w585, y=w586) -> (x*y=w584:dbl)
                            n134 = Add(x=w581, y=w584) -> (x+y=w583:dbl)
                          }
                          frame True {
                            n135 = Subtract(x=w594, y=w588) -> (x-y=w593:dbl)
                            n136 = Multiply(x=w592, y=w593) -> (x*y=w591:dbl)
                            n137 = Subtract(x=w590, y=w591) -> (x-y=w589:dbl)
                          }
                        }
                      }
                      frame True {
                        n138 = Multiply(x=w597, y=w598) -> (x*y=w596:dbl)
                        n139 = Add(x=w599, y=w596) -> (x+y=w595:dbl)
                      }
                    }
                    n140 = Absolute Value(x=w408) -> (abs(x)=w407:dbl)
                    n141 = stacked-sequence {
                      tunnel: w407 -> [w418 _ _ _]
                      tunnel: [_ _ w448 _] -> w403
                      tunnel: [_ _ w436 _] -> w394
                      tunnel: [_ _ _ w557] -> w402
                      tunnel: w401 -> [_ _ _ w556]
                      tunnel: [_ _ _ w555] -> w400
                      tunnel: w399 -> [_ _ _ w554]
                      tunnel: [_ _ _ w533] -> w398
                      tunnel: w397 -> [_ _ _ w553]
                      tunnel: [_ _ _ w552] -> w396
                      tunnel: w395 -> [_ _ _ w551]
                      tunnel: [_ _ w435 _] -> w393
                      tunnel: [_ _ w434 _] -> w389
                      tunnel: [_ _ w433 _] -> w392
                      tunnel: [_ _ w432 _] -> w391
                      tunnel: [_ _ w431 _] -> w390
                      tunnel: [_ _ w430 _] -> w388
                      tunnel: [_ _ w429 _] -> w387
                      tunnel: [_ _ w428 _] -> w386
                      tunnel: [_ _ w427 _] -> w385
                      tunnel: [_ _ _ w537] -> w384
                      tunnel: w383 -> [_ _ _ w536]
                      tunnel: [_ _ _ w535] -> w382
                      tunnel: w381 -> [_ _ _ w534]
                      frame #0 {
                        n142 = Format Into String(format string="SLVLD1,%.3f;", w418) -> (resulting string=w419:string)  [unwired: 2 in, 1 out]
                        n143 = local read "LOCKIN1 address"() -> (w417:refnum<visa-resource-name>)
                        n144 = Concatenate Strings(w419, "\r") -> (w415:string)
                        n145 = VISA Write(VISA resource name=w417, write buffer=w415) -> ()  [unwired: 1 in, 3 out]
                        n146 = local read "Two Channels ?"() -> (w416:bool)
                        n147 = case shown="True" w416 {
                          tunnel: w415 -> [_ w423]
                          frame False {
                          }
                          frame True {
                            n148 = local read "LOCKIN2 address"() -> (w422:refnum<visa-resource-name>)
                            n149 = VISA Write(VISA resource name=w422, write buffer=w423) -> ()  [unwired: 1 in, 3 out]
                          }
                        }
                        "Sine voltage T" <- w418
                      }
                      frame #1 {
                        n150 = local read "System Stablization (s)"() -> (w424:dbl)
                        n151 = Multiply(x=w424, y=1000) -> (x*y=w426:dbl)
                        n152 = Wait (ms)(milliseconds to wait=w426) -> ()  [unwired: 1 out]
                      }
                      frame #2 {
                        n153 = local read "LOCKIN1 address"() -> (w437:refnum<visa-resource-name>)
                        n154 = local read "Two Channels ?"() -> (w446:bool)
                        n155 = local read "LOCKIN2 address"() -> (w447:refnum<visa-resource-name>)
                        n156 = case shown="True" w446 {
                          tunnel: w447 -> [_ w497]
                          tunnel: [w484 w488] -> w430
                          tunnel: [w484 w487] -> w429
                          tunnel: [w484 w486] -> w428
                          tunnel: [w484 w485] -> w427
                          frame False {
                            w484 = nan
                          }
                          frame True {
                            n157 = flat-sequence {
                              tunnel: w497 -> [w511]
                              tunnel: [w510] -> w495
                              tunnel: [w509] -> w494
                              tunnel: [w508] -> w491
                              tunnel: [w507] -> w489
                              tunnel: [w499] -> w488
                              tunnel: [w498] -> w486
                              tunnel: [w520] -> w496
                              tunnel: w495 -> [w520]
                              tunnel: w494 -> [w519]
                              tunnel: [w519] -> w493
                              tunnel: [w518] -> w492
                              tunnel: w491 -> [w518]
                              tunnel: [w517] -> w490
                              tunnel: w489 -> [w517]
                              tunnel: w496 -> [w531]
                              tunnel: w493 -> [w530]
                              tunnel: w492 -> [w529]
                              tunnel: w490 -> [w528]
                              tunnel: [w523] -> w487
                              tunnel: [w522] -> w485
                              frame #0 {
                                w504 = u16 2 items=["X", "Y", "R", "Theta", "Frequency", "Noise", "Xh1", "Yh1", "Rh1", "Theta h1", "Xh2", "Yh2", "Rh2", "Theta h2"] ("Parameter 2")
                                w505 = u16 2 items=["X", "Y", "R", "Theta", "Frequency", "Noise", "Xh1", "Yh1", "Rh1", "Theta h1", "Xh2", "Yh2", "Rh2", "Theta h2"] ("Parameter")
                                w506 = u16 1 items=["Channel A", "Channel B", "ADC"] ("Channel (0: A)")
                                w512 = u16 0 items=["Channel A", "Channel B", "ADC"] ("Channel (0: A)")
                                n158 = Format Into String(0) -> (error out=w514:errorcluster)  [unwired: 3 in, 1 out]
                                n159 = Format Into String(0) -> (error out=w513:errorcluster)  [unwired: 3 in, 1 out]
                                n160 = call "OE1022D_Read 1 parameter_mean.vi"("错误输入（无错误）"=w514, "Parameter"=w505, "Channel (0: A)"=w512, "VISA resource name"=w511) -> ("error out"=w509:errorcluster, "Measurement"=w503:dbl, "VISA resource name out"=w510:refnum<visa-resource-name>)  [unwired: 5 in]
                                n161 = call "OE1022D_Read 1 parameter_mean.vi"("Parameter 2"=w504, "错误输入（无错误）"=w513, "Channel (0: A)"=w506, "VISA resource name"=w511) -> ("error out"=w507:errorcluster, "Measurement"=w502:dbl, "VISA resource name out"=w508:refnum<visa-resource-name>)  [unwired: 5 in]
                                n162 = local read "R2(Kohm)"() -> (w500:dbl)
                                n163 = Multiply(x=w502, y=1000.0) -> (x*y=w498:dbl)
                                n164 = Divide(x=w503, y=w500) -> (x/y=w499:dbl)
                              }
                              frame #1 {
                                n165 = Wait (ms)(milliseconds to wait=u32 50) -> ()  [unwired: 1 out]
                              }
                              frame #2 {
                                w524 = u16 3 items=["X", "Y", "R", "Theta", "Frequency", "Noise", "Xh1", "Yh1", "Rh1", "Theta h1", "Xh2", "Yh2", "Rh2", "Theta h2"] ("Parameter 2")
                                w525 = u16 1 items=["Channel A", "Channel B", "ADC"] ("Channel (0: A)")
                                w526 = u16 3 items=["X", "Y", "R", "Theta", "Frequency", "Noise", "Xh1", "Yh1", "Rh1", "Theta h1", "Xh2", "Yh2", "Rh2", "Theta h2"] ("Parameter")
                                w527 = u16 0 items=["Channel A", "Channel B", "ADC"] ("Channel (0: A)")
                                n166 = call "OE1022D_Read 1 parameter_mean.vi"("错误输入（无错误）"=w530, "Parameter"=w526, "Channel (0: A)"=w527, "VISA resource name"=w531) -> ("Measurement"=w523:dbl)  [unwired: 5 in, 2 out]
                                n167 = call "OE1022D_Read 1 parameter_mean.vi"("Parameter 2"=w524, "错误输入（无错误）"=w528, "Channel (0: A)"=w525, "VISA resource name"=w529) -> ("Measurement"=w522:dbl)  [unwired: 5 in, 2 out]
                              }
                              frame #3 {
                                n168 = Wait (ms)(milliseconds to wait=u32 50) -> ()  [unwired: 1 out]
                              }
                            }
                          }
                        }
                        "Ch2 Current(mA)" <- w430
                        "Ch 2 phase" <- w429
                        "Hall Voltage2(mV)" <- w428
                        "Hall Voltage 2 phase" <- w427
                        n169 = flat-sequence {
                          tunnel: w437 -> [w462]
                          tunnel: [w461] -> w445
                          tunnel: [w460] -> w444
                          tunnel: [w459] -> w443
                          tunnel: [w458] -> w442
                          tunnel: [w450] -> w433
                          tunnel: [w449] -> w431
                          tunnel: [w471] -> w441
                          tunnel: w445 -> [w471]
                          tunnel: w444 -> [w470]
                          tunnel: [w470] -> w440
                          tunnel: [w469] -> w439
                          tunnel: w443 -> [w469]
                          tunnel: [w468] -> w438
                          tunnel: w442 -> [w468]
                          tunnel: w441 -> [w482]
                          tunnel: w440 -> [w481]
                          tunnel: w439 -> [w480]
                          tunnel: w438 -> [w479]
                          tunnel: [w474] -> w432
                          tunnel: [w473] -> w434
                          frame #0 {
                            w455 = u16 2 items=["X", "Y", "R", "Theta", "Frequency", "Noise", "Xh1", "Yh1", "Rh1", "Theta h1", "Xh2", "Yh2", "Rh2", "Theta h2"] ("Parameter 2")
                            w456 = u16 2 items=["X", "Y", "R", "Theta", "Frequency", "Noise", "Xh1", "Yh1", "Rh1", "Theta h1", "Xh2", "Yh2", "Rh2", "Theta h2"] ("Parameter")
                            w457 = u16 1 items=["Channel A", "Channel B", "ADC"] ("Channel (0: A)")
                            w463 = u16 0 items=["Channel A", "Channel B", "ADC"] ("Channel (0: A)")
                            n170 = Format Into String(0) -> (error out=w465:errorcluster)  [unwired: 3 in, 1 out]
                            n171 = Format Into String(0) -> (error out=w464:errorcluster)  [unwired: 3 in, 1 out]
                            n172 = call "OE1022D_Read 1 parameter_mean.vi"("错误输入（无错误）"=w465, "Parameter"=w456, "Channel (0: A)"=w463, "VISA resource name"=w462) -> ("error out"=w460:errorcluster, "Measurement"=w454:dbl, "VISA resource name out"=w461:refnum<visa-resource-name>)  [unwired: 5 in]
                            n173 = call "OE1022D_Read 1 parameter_mean.vi"("Parameter 2"=w455, "错误输入（无错误）"=w464, "Channel (0: A)"=w457, "VISA resource name"=w462) -> ("error out"=w458:errorcluster, "Measurement"=w453:dbl, "VISA resource name out"=w459:refnum<visa-resource-name>)  [unwired: 5 in]
                            n174 = local read "R1(Kohm)"() -> (w451:dbl)
                            n175 = Multiply(x=w453, y=1000.0) -> (x*y=w449:dbl)
                            n176 = Divide(x=w454, y=w451) -> (x/y=w450:dbl)
                          }
                          frame #1 {
                            n177 = Wait (ms)(milliseconds to wait=u32 50) -> ()  [unwired: 1 out]
                          }
                          frame #2 {
                            w475 = u16 3 items=["X", "Y", "R", "Theta", "Frequency", "Noise", "Xh1", "Yh1", "Rh1", "Theta h1", "Xh2", "Yh2", "Rh2", "Theta h2"] ("Parameter 2")
                            w476 = u16 1 items=["Channel A", "Channel B", "ADC"] ("Channel (0: A)")
                            w477 = u16 3 items=["X", "Y", "R", "Theta", "Frequency", "Noise", "Xh1", "Yh1", "Rh1", "Theta h1", "Xh2", "Yh2", "Rh2", "Theta h2"] ("Parameter")
                            w478 = u16 0 items=["Channel A", "Channel B", "ADC"] ("Channel (0: A)")
                            n178 = call "OE1022D_Read 1 parameter_mean.vi"("错误输入（无错误）"=w481, "Parameter"=w477, "Channel (0: A)"=w478, "VISA resource name"=w482) -> ("Measurement"=w474:dbl)  [unwired: 5 in, 2 out]
                            n179 = call "OE1022D_Read 1 parameter_mean.vi"("Parameter 2"=w475, "错误输入（无错误）"=w479, "Channel (0: A)"=w476, "VISA resource name"=w480) -> ("Measurement"=w473:dbl)  [unwired: 5 in, 2 out]
                          }
                          frame #3 {
                            n180 = Wait (ms)(milliseconds to wait=u32 50) -> ()  [unwired: 1 out]
                          }
                        }
                        n181 = local read "Temperature"() -> (w436:dbl)
                        n182 = local read "Sine voltage T"() -> (w448:dbl)
                        n183 = local read "Field"() -> (w435:dbl)
                        "Ch1 Current(mA)" <- w433
                        "Ch 1 phase" <- w432
                        "Hall Voltage1(mV)" <- w431
                        "Hall Voltage 1 phase" <- w434
                      }
                      frame #3 {
                        n184 = local read "Ch1 Current(mA)"() -> (w558:dbl)
                        n185 = local read "Ch2 Current(mA)"() -> (w547:dbl)
                        n186 = local read "Hall Voltage2(mV)"() -> (w546:dbl)
                        n187 = Build Array (concatenate)(w558, w536) -> (w537:dbl[])
                        n188 = Build Array (concatenate)(w547, w534) -> (w535:dbl[])
                        n189 = local read "Hall Voltage1(mV)"() -> (w550:dbl)
                        n190 = Build Array(w546) -> (w569:dbl[])
                        n191 = Build Array(w550) -> (w570:dbl[])
                        n192 = Select(t=w569, s="Ch2 Plot Clear", f=w553) -> (s? t:f=w559:dbl[])
                        n193 = Select(t=w570, s="Ch1 Plot Clear", f=w556) -> (s? t:f=w566:dbl[])
                        n194 = Build Array (concatenate)(w546, w559) -> (w533:dbl[])
                        n195 = Build Array (concatenate)(w550, w566) -> (w557:dbl[])
                        n196 = Bundle(w535, w533) -> (→"Hall Voltage 2":cluster{dbl[], dbl[]})  [unwired: 1 in]
                        n197 = Bundle(w537, w557) -> (→"Hall Voltage 1":cluster{dbl[], dbl[]})  [unwired: 1 in]
                        n198 = local read "Hall Voltage 2 phase"() -> (w540:dbl)
                        n199 = local read "Hall Voltage 1 phase"() -> (w542:dbl)
                        n200 = local read "Ch 2 phase"() -> (w539:dbl)
                        n201 = local read "Ch 1 phase"() -> (w543:dbl)
                        n202 = Subtract(x=w540, y=w539) -> (x-y=w541:dbl)
                        n203 = Subtract(x=w542, y=w543) -> (x-y=w545:dbl)
                        n204 = Absolute Value(x=w541) -> (abs(x)=w538:dbl)
                        n205 = Absolute Value(x=w545) -> (abs(x)=w544:dbl)
                        n206 = Build Array(w544) -> (w565:dbl[])
                        n207 = Build Array(w538) -> (w562:dbl[])
                        n208 = Select(t=w565, s="Ch1 Plot Clear", f=w554) -> (s? t:f=w563:dbl[])
                        n209 = Select(t=w562, s="Ch2 Plot Clear", f=w551) -> (s? t:f=w560:dbl[])
                        n210 = Build Array (concatenate)(w544, w563) -> (w555:dbl[])
                        n211 = Build Array (concatenate)(w538, w560) -> (w552:dbl[])
                        n212 = Bundle(w537, w555) -> (→"Hall Voltage 1 reletive phase":cluster{dbl[], dbl[]})  [unwired: 1 in]
                        n213 = Bundle(w535, w552) -> (→"Hall Voltage 2 reletive phase":cluster{dbl[], dbl[]})  [unwired: 1 in]
                      }
                    }
                    n214 = case shown="True" w406 {
                      tunnel: w403 -> [_ w604]
                      tunnel: w405 -> [_ w612]
                      tunnel: w404 -> [_ w611]
                      tunnel: w394 -> [_ w606]
                      tunnel: w393 -> [_ w605]
                      tunnel: w392 -> [_ w610]
                      tunnel: w391 -> [_ w609]
                      tunnel: w390 -> [_ w608]
                      tunnel: w389 -> [_ w607]
                      tunnel: w388 -> [_ w603]
                      tunnel: w387 -> [_ w602]
                      tunnel: w386 -> [_ w601]
                      tunnel: w385 -> [_ w600]
                      frame False {
                      }
                      frame True {
                        n215 = Build Array(w606, w605, w604, w610, w609, w608, w607) -> (w615:dbl[])
                        n216 = local read "Two Channels ?"() -> (w613:bool)
                        n217 = call-poly <vilib>:"Write Delimited Spreadsheet.vi"("file path (dialog if empty)"=w612, "format (%.3f)"="%.10f", "1D data"=w615, "append to file? (new file:F)"=TRUE) -> ()  [unwired: 10 in, 2 out]
                        n218 = case shown="True" w613 {
                          tunnel: w611 -> [_ w624]
                          tunnel: w606 -> [_ w623]
                          tunnel: w605 -> [_ w622]
                          tunnel: w604 -> [_ w621]
                          tunnel: w603 -> [_ w620]
                          tunnel: w602 -> [_ w619]
                          tunnel: w601 -> [_ w618]
                          tunnel: w600 -> [_ w617]
                          frame False {
                          }
                          frame True {
                            n219 = Build Array(w623, w622, w621, w620, w619, w618, w617) -> (w626:dbl[])
                            n220 = call-poly <vilib>:"Write Delimited Spreadsheet.vi"("file path (dialog if empty)"=w624, "format (%.3f)"="%.10f", "1D data"=w626, "append to file? (new file:F)"=TRUE) -> ()  [unwired: 10 in, 2 out]
                          }
                        }
                      }
                    }
                  }
                }
              }
              frame #4 {
                n221 = local read "FIxed F Rate (Oe/s)"() -> (w640:dbl)
                n222 = local read "FIxed F (Oe)"() -> (w642:dbl)
                n223 = local read "Fixed Field Approach"() -> (w638:i32)
                n224 = Negate(x=w642) -> (-x=w641:dbl)
                n225 = local read "Fixed F mode"() -> (w639:i32)
                n226 = local write "FIxed F (Oe)"(w641) -> ()
                n227 = call "SetField.vi"("Mode"=w639, "Approach"=w638, "Rate"=w640, "Field"=w641, "error in (no error)"=w628, "Instrument Ref In"=w629) -> ("error out"=w645:errorcluster, "Instrument Ref Out"=w646:refnum<k24>)  [unwired: 1 in, 1 out]
                n228 = local read "F Delay"() -> (w643:dbl)
                n229 = call "WaitFor.vi"("Delay"=w643, "Wait For Field"=TRUE, "error in (no error)"=w645, "Instrument Ref In"=w646) -> ("error out"=w633:errorcluster, "Instrument Ref Out"=w632:refnum<k24>)  [unwired: 6 in]
                n230 = for {
                  N: 20 -> [_]
                  shift-right: [w657] -> _
                  shift-left: TRUE -> [w655]
                  shift-right: [w652] -> _
                  shift-left: w633 -> [w654]
                  tunnel: w632 -> [w651]
                  tunnel: [w649] -> _
                  tunnel: [w647] -> w634 mode=indexing
                  tunnel: [w648] -> w635 mode=indexing
                  n231 = Not(x=w655) -> (.not. x?=w657:bool)
                  n232 = call "GetTemperature.vi"("error in (no error)"=w654, "Instrument Ref In"=w651) -> ("Temperature"=w648:dbl, "error out"=w653:errorcluster, "Instrument Ref Out"=w650:refnum<k24>)  [unwired: 3 in, 2 out]
                  n233 = local write "Measuring"(w655) -> ()
                  n234 = Wait (ms)(milliseconds to wait=u32 200) -> ()  [unwired: 1 out]
                  n235 = call "GetField.vi"("error in (no error)"=w653, "Instrument Ref In"=w650) -> ("Field"=w647:dbl, "error out"=w652:errorcluster, "Instrument Ref Out"=w649:refnum<k24>)  [unwired: 3 in, 2 out]
                }
                n236 = call-poly <vilib>:"Mean.vi"("X"=w634) -> ("mean"=w631:dbl)  [unwired: 1 out]
                n237 = call-poly <vilib>:"Mean.vi"("X"=w635) -> ("mean"=w630:dbl)  [unwired: 1 out]
                n238 = local write "Measured Temp (K)"(w630) -> ()
                n239 = local write "Measured Field (Oe)"(w631) -> ()
              }
              frame #5 {
                n240 = local read "V Loop#"() -> (w661:i32)
                n241 = for {
                  N: w661 -> [_]
                  tunnel: w660 -> [w673]
                  tunnel: w659 -> [w672]
                  tunnel: w658 -> [w671]
                  shift-right: [w670] -> _
                  shift-left: _ -> [w669]
                  shift-right: [w668] -> _
                  shift-left: _ -> [w667]
                  shift-right: [w666] -> _
                  shift-left: _ -> [w665]
                  shift-right: [w664] -> _
                  shift-left: _ -> [w663]
                  i -> [w685]
                  n242 = local read "V Step(mV)"() -> (w674:i32)
                  n243 = Add(x=1, y=w685) -> (x+y=w662:i32)
                  n244 = local read "High Value (V)"() -> (w676:dbl)
                  n245 = local read "Low Value (V)"() -> (w675:dbl)
                  n246 = local write "V Loop Run T"(w662) -> ()
                  n247 = Subtract(x=w676, y=w675) -> (x-y=w681:dbl)
                  n248 = Divide(x=w674, y=1000) -> (x/y=w678:dbl)
                  n249 = Divide(x=w681, y=w678) -> (x/y=w677:dbl)
                  n250 = Multiply(x=2, y=w677) -> (x*y=w680:dbl)
                  n251 = Increment(x=w680) -> (x+1=w679:dbl)
                  n252 = for {
                    N: w679 -> [_]
                    tunnel: w678 -> [w714]
                    tunnel: w677 -> [w716]
                    tunnel: w673 -> [w711]
                    tunnel: w672 -> [w710]
                    tunnel: w671 -> [w709]
                    shift-right: [w707] -> w670
                    shift-left: w669 -> [w706]
                    shift-right: [w705] -> w668
                    shift-left: w667 -> [w704]
                    shift-right: [w703] -> w666
                    shift-left: w665 -> [w702]
                    shift-right: [w701] -> w664
                    shift-left: w663 -> [w700]
                    shift-right: [w689] -> _
                    shift-left: _ -> [w688]
                    shift-right: [w687] -> _
                    shift-left: _ -> [w686]
                    i -> [w715]
                    n253 = local read "High Value (V)"() -> (w718:dbl)
                    n254 = local read "Low Value (V)"() -> (w719:dbl)
                    n255 = Less Or Equal?(x=w715, y=w716) -> (x <= y?=w717:bool)
                    n256 = case shown="False" w717 {
                      tunnel: w719 -> [w876 w904]
                      tunnel: w715 -> [w885 w903]
                      tunnel: w714 -> [w884 w902]
                      tunnel: [w882 w900] -> w713
                      tunnel: w718 -> [w883 _]
                      tunnel: w716 -> [w878 _]
                      tunnel: w715 -> [w881 _]
                      frame False {
                        n257 = Multiply(x=w878, y=2) -> (x*y=w877:dbl)
                        n258 = Less Or Equal?(x=w881, y=w877) -> (x <= y?=w879:bool)
                        n259 = case shown="False" w879 {
                          tunnel: w885 -> [w892 w899]
                          tunnel: w884 -> [w890 w897]
                          tunnel: w883 -> [_ w895]
                          tunnel: [w888 w894] -> w882
                          tunnel: w878 -> [_ w893]
                          tunnel: w877 -> [w887 _]
                          tunnel: w876 -> [w886 _]
                          frame False {
                            n260 = Subtract(x=w892, y=w887) -> (x-y=w891:dbl)
                            n261 = Multiply(x=w890, y=w891) -> (x*y=w889:dbl)
                            n262 = Add(x=w886, y=w889) -> (x+y=w888:dbl)
                          }
                          frame True {
                            n263 = Subtract(x=w899, y=w893) -> (x-y=w898:dbl)
                            n264 = Multiply(x=w897, y=w898) -> (x*y=w896:dbl)
                            n265 = Subtract(x=w895, y=w896) -> (x-y=w894:dbl)
                          }
                        }
                      }
                      frame True {
                        n266 = Multiply(x=w902, y=w903) -> (x*y=w901:dbl)
                        n267 = Add(x=w904, y=w901) -> (x+y=w900:dbl)
                      }
                    }
                    n268 = Absolute Value(x=w713) -> (abs(x)=w712:dbl)
                    n269 = stacked-sequence {
                      tunnel: w712 -> [w720 _ _ _]
                      tunnel: [_ _ w753 _] -> w708
                      tunnel: [_ _ w741 _] -> w699
                      tunnel: [_ _ _ w866] -> w707
                      tunnel: w706 -> [_ _ _ w865]
                      tunnel: [_ _ _ w864] -> w705
                      tunnel: w704 -> [_ _ _ w863]
                      tunnel: [_ _ _ w844] -> w703
                      tunnel: w702 -> [_ _ _ w862]
                      tunnel: [_ _ _ w861] -> w701
                      tunnel: w700 -> [_ _ _ w860]
                      tunnel: [_ _ w740 _] -> w698
                      tunnel: [_ _ w736 _] -> w694
                      tunnel: [_ _ w739 _] -> w697
                      tunnel: [_ _ w738 _] -> w696
                      tunnel: [_ _ w737 _] -> w695
                      tunnel: [_ _ w735 _] -> w693
                      tunnel: [_ _ w734 _] -> w692
                      tunnel: [_ _ w733 _] -> w691
                      tunnel: [_ _ w732 _] -> w690
                      tunnel: [_ _ _ w848] -> w689
                      tunnel: w688 -> [_ _ _ w847]
                      tunnel: [_ _ _ w846] -> w687
                      tunnel: w686 -> [_ _ _ w845]
                      frame #0 {
                        n270 = local write "Sine voltage T"(w720) -> ()
                        n271 = Format Into String(format string="SLVLD1,%.3f;", w720) -> (resulting string=w724:string)  [unwired: 2 in, 1 out]
                        n272 = local read "LOCKIN1 address"() -> (w723:refnum<visa-resource-name>)
                        n273 = Concatenate Strings(w724, "\r") -> (w721:string)
                        n274 = VISA Write(VISA resource name=w723, write buffer=w721) -> ()  [unwired: 1 in, 3 out]
                        n275 = local read "Two Channels ?"() -> (w722:bool)
                        n276 = case shown="False" w722 {
                          tunnel: w721 -> [_ w728]
                          frame False {
                          }
                          frame True {
                            n277 = local read "LOCKIN2 address"() -> (w727:refnum<visa-resource-name>)
                            n278 = VISA Write(VISA resource name=w727, write buffer=w728) -> ()  [unwired: 1 in, 3 out]
                          }
                        }
                      }
                      frame #1 {
                        n279 = local read "System Stablization (s)"() -> (w729:dbl)
                        n280 = Multiply(x=w729, y=1000) -> (x*y=w731:dbl)
                        n281 = Wait (ms)(milliseconds to wait=w731) -> ()  [unwired: 1 out]
                      }
                      frame #2 {
                        n282 = local read "LOCKIN1 address"() -> (w742:refnum<visa-resource-name>)
                        n283 = local read "Two Channels ?"() -> (w751:bool)
                        n284 = local read "LOCKIN2 address"() -> (w752:refnum<visa-resource-name>)
                        n285 = case shown="True" w751 {
                          tunnel: w752 -> [_ w802]
                          tunnel: [w789 w793] -> w735
                          tunnel: [w789 w792] -> w734
                          tunnel: [w789 w791] -> w733
                          tunnel: [w789 w790] -> w732
                          frame False {
                            w789 = nan
                          }
                          frame True {
                            n286 = flat-sequence {
                              tunnel: w802 -> [w816]
                              tunnel: [w815] -> w800
                              tunnel: [w814] -> w799
                              tunnel: [w813] -> w796
                              tunnel: [w812] -> w794
                              tunnel: [w804] -> w793
                              tunnel: [w803] -> w791
                              tunnel: [w825] -> w801
                              tunnel: w800 -> [w825]
                              tunnel: w799 -> [w824]
                              tunnel: [w824] -> w798
                              tunnel: [w823] -> w797
                              tunnel: w796 -> [w823]
                              tunnel: [w822] -> w795
                              tunnel: w794 -> [w822]
                              tunnel: w801 -> [w836]
                              tunnel: w798 -> [w835]
                              tunnel: w797 -> [w834]
                              tunnel: w795 -> [w833]
                              tunnel: [w828] -> w792
                              tunnel: [w827] -> w790
                              frame #0 {
                                w809 = u16 2 items=["X", "Y", "R", "Theta", "Frequency", "Noise", "Xh1", "Yh1", "Rh1", "Theta h1", "Xh2", "Yh2", "Rh2", "Theta h2"] ("Parameter 2")
                                w810 = u16 2 items=["X", "Y", "R", "Theta", "Frequency", "Noise", "Xh1", "Yh1", "Rh1", "Theta h1", "Xh2", "Yh2", "Rh2", "Theta h2"] ("Parameter")
                                w811 = u16 1 items=["Channel A", "Channel B", "ADC"] ("Channel (0: A)")
                                w817 = u16 0 items=["Channel A", "Channel B", "ADC"] ("Channel (0: A)")
                                n287 = Format Into String(0) -> (error out=w819:errorcluster)  [unwired: 3 in, 1 out]
                                n288 = Format Into String(0) -> (error out=w818:errorcluster)  [unwired: 3 in, 1 out]
                                n289 = call "OE1022D_Read 1 parameter_mean.vi"("错误输入（无错误）"=w819, "Parameter"=w810, "Channel (0: A)"=w817, "VISA resource name"=w816) -> ("error out"=w814:errorcluster, "Measurement"=w808:dbl, "VISA resource name out"=w815:refnum<visa-resource-name>)  [unwired: 5 in]
                                n290 = call "OE1022D_Read 1 parameter_mean.vi"("Parameter 2"=w809, "错误输入（无错误）"=w818, "Channel (0: A)"=w811, "VISA resource name"=w816) -> ("error out"=w812:errorcluster, "Measurement"=w807:dbl, "VISA resource name out"=w813:refnum<visa-resource-name>)  [unwired: 5 in]
                                n291 = local read "R2(Kohm)"() -> (w805:dbl)
                                n292 = Multiply(x=w807, y=1000.0) -> (x*y=w803:dbl)
                                n293 = Divide(x=w808, y=w805) -> (x/y=w804:dbl)
                              }
                              frame #1 {
                                n294 = Wait (ms)(milliseconds to wait=u32 50) -> ()  [unwired: 1 out]
                              }
                              frame #2 {
                                w829 = u16 3 items=["X", "Y", "R", "Theta", "Frequency", "Noise", "Xh1", "Yh1", "Rh1", "Theta h1", "Xh2", "Yh2", "Rh2", "Theta h2"] ("Parameter 2")
                                w830 = u16 1 items=["Channel A", "Channel B", "ADC"] ("Channel (0: A)")
                                w831 = u16 3 items=["X", "Y", "R", "Theta", "Frequency", "Noise", "Xh1", "Yh1", "Rh1", "Theta h1", "Xh2", "Yh2", "Rh2", "Theta h2"] ("Parameter")
                                w832 = u16 0 items=["Channel A", "Channel B", "ADC"] ("Channel (0: A)")
                                n295 = call "OE1022D_Read 1 parameter_mean.vi"("错误输入（无错误）"=w835, "Parameter"=w831, "Channel (0: A)"=w832, "VISA resource name"=w836) -> ("Measurement"=w828:dbl)  [unwired: 5 in, 2 out]
                                n296 = call "OE1022D_Read 1 parameter_mean.vi"("Parameter 2"=w829, "错误输入（无错误）"=w833, "Channel (0: A)"=w830, "VISA resource name"=w834) -> ("Measurement"=w827:dbl)  [unwired: 5 in, 2 out]
                              }
                              frame #3 {
                                n297 = Wait (ms)(milliseconds to wait=u32 50) -> ()  [unwired: 1 out]
                              }
                            }
                          }
                        }
                        n298 = flat-sequence {
                          tunnel: w742 -> [w767]
                          tunnel: [w766] -> w750
                          tunnel: [w765] -> w749
                          tunnel: [w764] -> w748
                          tunnel: [w763] -> w747
                          tunnel: [w755] -> w739
                          tunnel: [w754] -> w737
                          tunnel: [w776] -> w746
                          tunnel: w750 -> [w776]
                          tunnel: w749 -> [w775]
                          tunnel: [w775] -> w745
                          tunnel: [w774] -> w744
                          tunnel: w748 -> [w774]
                          tunnel: [w773] -> w743
                          tunnel: w747 -> [w773]
                          tunnel: w746 -> [w787]
                          tunnel: w745 -> [w786]
                          tunnel: w744 -> [w785]
                          tunnel: w743 -> [w784]
                          tunnel: [w779] -> w738
                          tunnel: [w778] -> w736
                          frame #0 {
                            w760 = u16 2 items=["X", "Y", "R", "Theta", "Frequency", "Noise", "Xh1", "Yh1", "Rh1", "Theta h1", "Xh2", "Yh2", "Rh2", "Theta h2"] ("Parameter 2")
                            w761 = u16 2 items=["X", "Y", "R", "Theta", "Frequency", "Noise", "Xh1", "Yh1", "Rh1", "Theta h1", "Xh2", "Yh2", "Rh2", "Theta h2"] ("Parameter")
                            w762 = u16 1 items=["Channel A", "Channel B", "ADC"] ("Channel (0: A)")
                            w768 = u16 0 items=["Channel A", "Channel B", "ADC"] ("Channel (0: A)")
                            n299 = Format Into String(0) -> (error out=w770:errorcluster)  [unwired: 3 in, 1 out]
                            n300 = Format Into String(0) -> (error out=w769:errorcluster)  [unwired: 3 in, 1 out]
                            n301 = call "OE1022D_Read 1 parameter_mean.vi"("错误输入（无错误）"=w770, "Parameter"=w761, "Channel (0: A)"=w768, "VISA resource name"=w767) -> ("error out"=w765:errorcluster, "Measurement"=w759:dbl, "VISA resource name out"=w766:refnum<visa-resource-name>)  [unwired: 5 in]
                            n302 = call "OE1022D_Read 1 parameter_mean.vi"("Parameter 2"=w760, "错误输入（无错误）"=w769, "Channel (0: A)"=w762, "VISA resource name"=w767) -> ("error out"=w763:errorcluster, "Measurement"=w758:dbl, "VISA resource name out"=w764:refnum<visa-resource-name>)  [unwired: 5 in]
                            n303 = local read "R1(Kohm)"() -> (w756:dbl)
                            n304 = Multiply(x=w758, y=1000.0) -> (x*y=w754:dbl)
                            n305 = Divide(x=w759, y=w756) -> (x/y=w755:dbl)
                          }
                          frame #1 {
                            n306 = Wait (ms)(milliseconds to wait=u32 50) -> ()  [unwired: 1 out]
                          }
                          frame #2 {
                            w780 = u16 3 items=["X", "Y", "R", "Theta", "Frequency", "Noise", "Xh1", "Yh1", "Rh1", "Theta h1", "Xh2", "Yh2", "Rh2", "Theta h2"] ("Parameter 2")
                            w781 = u16 1 items=["Channel A", "Channel B", "ADC"] ("Channel (0: A)")
                            w782 = u16 3 items=["X", "Y", "R", "Theta", "Frequency", "Noise", "Xh1", "Yh1", "Rh1", "Theta h1", "Xh2", "Yh2", "Rh2", "Theta h2"] ("Parameter")
                            w783 = u16 0 items=["Channel A", "Channel B", "ADC"] ("Channel (0: A)")
                            n307 = call "OE1022D_Read 1 parameter_mean.vi"("错误输入（无错误）"=w786, "Parameter"=w782, "Channel (0: A)"=w783, "VISA resource name"=w787) -> ("Measurement"=w779:dbl)  [unwired: 5 in, 2 out]
                            n308 = call "OE1022D_Read 1 parameter_mean.vi"("Parameter 2"=w780, "错误输入（无错误）"=w784, "Channel (0: A)"=w781, "VISA resource name"=w785) -> ("Measurement"=w778:dbl)  [unwired: 5 in, 2 out]
                          }
                          frame #3 {
                            n309 = Wait (ms)(milliseconds to wait=u32 50) -> ()  [unwired: 1 out]
                          }
                        }
                        n310 = local read "Temperature"() -> (w741:dbl)
                        n311 = local read "FIxed F (Oe)"() -> (w740:dbl)
                        n312 = local read "Sine voltage T"() -> (w753:dbl)
                        n313 = local write "Ch1 Current(mA)"(w739) -> ()
                        n314 = local write "Hall Voltage 1 phase"(w736) -> ()
                        n315 = local write "Hall Voltage 2 phase"(w732) -> ()
                        n316 = local write "Hall Voltage1(mV)"(w737) -> ()
                        n317 = local write "Hall Voltage2(mV)"(w733) -> ()
                        n318 = local write "Ch 1 phase"(w738) -> ()
                        n319 = local write "Ch2 Current(mA)"(w735) -> ()
                        n320 = local write "Ch 2 phase"(w734) -> ()
                      }
                      frame #3 {
                        n321 = local read "Ch1 Current(mA)"() -> (w867:dbl)
                        n322 = local read "Ch2 Current(mA)"() -> (w858:dbl)
                        n323 = local read "Hall Voltage2(mV)"() -> (w857:dbl)
                        n324 = Build Array (concatenate)(w867, w847) -> (w848:dbl[])
                        n325 = Build Array (concatenate)(w858, w845) -> (w846:dbl[])
                        n326 = local read "Hall Voltage1(mV)"() -> (w859:dbl)
                        n327 = local read "Ch1 Plot Clear"() -> (w839:bool)
                        n328 = local read "Ch2 Plot Clear"() -> (w838:bool)
                        n329 = Build Array(w857) -> (w874:dbl[])
                        n330 = Build Array(w859) -> (w875:dbl[])
                        n331 = Select(t=w874, s=w838, f=w862) -> (s? t:f=w868:dbl[])
                        n332 = Select(t=w875, s=w839, f=w865) -> (s? t:f=w873:dbl[])
                        n333 = Build Array (concatenate)(w857, w868) -> (w844:dbl[])
                        n334 = Build Array (concatenate)(w859, w873) -> (w866:dbl[])
                        n335 = Bundle(w846, w844) -> (w840:cluster{dbl[], dbl[]})  [unwired: 1 in]
                        n336 = Bundle(w848, w866) -> (w843:cluster{dbl[], dbl[]})  [unwired: 1 in]
                        n337 = local write "Hall Voltage 1"(w843) -> ()
                        n338 = local write "Hall Voltage 2"(w840) -> ()
                        n339 = local read "Hall Voltage 2 phase"() -> (w851:dbl)
                        n340 = local read "Hall Voltage 1 phase"() -> (w853:dbl)
                        n341 = local read "Ch 2 phase"() -> (w850:dbl)
                        n342 = local read "Ch 1 phase"() -> (w854:dbl)
                        n343 = Subtract(x=w851, y=w850) -> (x-y=w852:dbl)
                        n344 = Subtract(x=w853, y=w854) -> (x-y=w856:dbl)
                        n345 = Absolute Value(x=w852) -> (abs(x)=w849:dbl)
                        n346 = Absolute Value(x=w856) -> (abs(x)=w855:dbl)
                        n347 = Build Array(w855) -> (w872:dbl[])
                        n348 = Build Array(w849) -> (w870:dbl[])
                        n349 = Select(t=w872, s=w839, f=w863) -> (s? t:f=w871:dbl[])
                        n350 = Select(t=w870, s=w838, f=w860) -> (s? t:f=w869:dbl[])
                        n351 = Build Array (concatenate)(w855, w871) -> (w864:dbl[])
                        n352 = Build Array (concatenate)(w849, w869) -> (w861:dbl[])
                        n353 = Bundle(w848, w864) -> (w842:cluster{dbl[], dbl[]})  [unwired: 1 in]
                        n354 = Bundle(w846, w861) -> (w841:cluster{dbl[], dbl[]})  [unwired: 1 in]
                        n355 = local write "Hall Voltage 1 reletive phase"(w842) -> ()
                        n356 = local write "Hall Voltage 2 reletive phase"(w841) -> ()
                      }
                    }
                    n357 = case shown="True" w711 {
                      tunnel: w708 -> [_ w909]
                      tunnel: w710 -> [_ w917]
                      tunnel: w709 -> [_ w916]
                      tunnel: w699 -> [_ w911]
                      tunnel: w698 -> [_ w910]
                      tunnel: w697 -> [_ w915]
                      tunnel: w696 -> [_ w914]
                      tunnel: w695 -> [_ w913]
                      tunnel: w694 -> [_ w912]
                      tunnel: w693 -> [_ w908]
                      tunnel: w692 -> [_ w907]
                      tunnel: w691 -> [_ w906]
                      tunnel: w690 -> [_ w905]
                      frame False {
                      }
                      frame True {
                        n358 = Build Array(w911, w910, w909, w915, w914, w913, w912) -> (w920:dbl[])
                        n359 = local read "Two Channels ?"() -> (w918:bool)
                        n360 = call-poly <vilib>:"Write Delimited Spreadsheet.vi"("file path (dialog if empty)"=w917, "format (%.3f)"="%.10f", "1D data"=w920, "append to file? (new file:F)"=TRUE) -> ()  [unwired: 10 in, 2 out]
                        n361 = case shown="True" w918 {
                          tunnel: w916 -> [_ w929]
                          tunnel: w911 -> [_ w928]
                          tunnel: w910 -> [_ w927]
                          tunnel: w909 -> [_ w926]
                          tunnel: w908 -> [_ w925]
                          tunnel: w907 -> [_ w924]
                          tunnel: w906 -> [_ w923]
                          tunnel: w905 -> [_ w922]
                          frame False {
                          }
                          frame True {
                            n362 = Build Array(w928, w927, w926, w925, w924, w923, w922) -> (w931:dbl[])
                            n363 = call-poly <vilib>:"Write Delimited Spreadsheet.vi"("file path (dialog if empty)"=w929, "format (%.3f)"="%.10f", "1D data"=w931, "append to file? (new file:F)"=TRUE) -> ()  [unwired: 10 in, 2 out]
                          }
                        }
                      }
                    }
                  }
                }
              }
            }
          }
        }
      }
      "Forward" <- FALSE ("Up")
      "Backward" <- FALSE ("Down")
    }
    frame #2 {
      n364 = case shown="True" "Initialization?" {
        tunnel: w935 -> [w936 w939]
        tunnel: w934 -> [w937 w938]
        frame False {
          n365 = Close Reference(reference=w937, error in (no error)=w936) -> ()  [unwired: 1 out]
        }
        frame True {
          w945 = 0 items=["Linear", "NoOvershoot", "Oscillate"] ("Approach")
          w946 = 0 items=["Persistent", "Driven"] ("Mode")
          w942 = 0 items=["FastSettle", "NoOvershoot"] ("Approach")
          n366 = call "SetTemperature.vi"("Approach"=w942, "Rate"=20.0, "Temperature"=1.6, "error in (no error)"=w939, "Instrument Ref In"=w938) -> ("error out"=w950:errorcluster, "Instrument Ref Out"=w949:refnum<k24>)  [unwired: 2 in, 1 out]
          n367 = call "SetField.vi"("Mode"=w946, "Approach"=w945, "Rate"=200.0, "Field"=0.0, "error in (no error)"=w950, "Instrument Ref In"=w949) -> ("error out"=w947:errorcluster, "Instrument Ref Out"=w948:refnum<k24>)  [unwired: 1 in, 1 out]
          n368 = Close Reference(reference=w948, error in (no error)=w947) -> ()  [unwired: 1 out]
        }
      }
    }
  }
  n369 = while {
    tunnel: w32 -> [w953]
    tunnel: w31 -> [w952]
    stop <- "?" stop-if-true
    n370 = for {
      N: 10 -> [_]
      shift-right: [w968] -> _
      shift-left: w952 -> [w970]
      tunnel: w953 -> [w967]
      tunnel: [w965] -> _
      tunnel: [w962] -> w959
      tunnel: [w961] -> w958
      tunnel: [w963] -> w956 mode=indexing
      tunnel: [w964] -> w957 mode=indexing
      n371 = call "GetTemperature.vi"("error in (no error)"=w970, "Instrument Ref In"=w967) -> ("Temperature\nStatus"=w961:i32, "Temperature"=w964:dbl, "error out"=w969:errorcluster, "Instrument Ref Out"=w966:refnum<k24>)  [unwired: 3 in, 1 out]
      n372 = Wait (ms)(milliseconds to wait=u32 200) -> ()  [unwired: 1 out]
      n373 = call "GetField.vi"("error in (no error)"=w969, "Instrument Ref In"=w966) -> ("Field\nStatus"=w962:i32, "Field"=w963:dbl, "error out"=w968:errorcluster, "Instrument Ref Out"=w965:refnum<k24>)  [unwired: 3 in, 1 out]
    }
    "Field Status" <- w959
    "Temperature Status" <- w958
    n374 = call-poly <vilib>:"Mean.vi"("X"=w956) -> ("mean"=→"Field":dbl)  [unwired: 1 out]
    n375 = call-poly <vilib>:"Mean.vi"("X"=w957) -> ("mean"=→"Temperature":dbl)  [unwired: 1 out]
  }
  n376 = local read "Start Value (K)"() -> (w2:dbl)
  n377 = local read "End Value (K)"() -> (w3:dbl)
  n378 = Format Into String(format string="%dKohm", "R1(Kohm)") -> (resulting string=w11:string)  [unwired: 2 in, 1 out]
  n379 = Format Into String(format string="%dK", initial string="to", w3) -> (resulting string=w21:string)  [unwired: 1 in, 1 out]
  n380 = Format Into String(format string="%.0fOe", initial string="at", "FIxed F (Oe)") -> (resulting string=w20:string)  [unwired: 1 in, 1 out]
  n381 = Format Into String(format string="%d", initial string="from", w2) -> (resulting string=w22:string)  [unwired: 1 in, 1 out]
  n382 = local read "Two Channels ?"() -> (w14:bool)
  n383 = case shown="False" w14 {
    tunnel: [w972 w974] -> w10
    tunnel: w11 -> [w972 w973]
    frame False {
    }
    frame True {
      n384 = Format Into String(format string="%dKohm", initial string=w973, "R2(Kohm)") -> (resulting string=w974:string)  [unwired: 1 in, 1 out]
    }
  }
  n385 = local read "A frequency"() -> (w27:dbl)
  n386 = Format Into String(format string="%dHz", initial string="at", w27) -> (resulting string=w19:string)  [unwired: 1 in, 1 out]
  n387 = Format Into String(initial string="path1 (folder + filename)", w23, w22, w21, w20, w19, w10, w18) -> (resulting string=w30:string)  [unwired: 2 in, 1 out]
  n388 = String To Path(string=w30) -> (path=w17:path)
  n389 = Format Into String(initial string="path2 (folder + filename)", w23, w22, w21, w20, w19, w10, w18) -> (resulting string=w29:string)  [unwired: 2 in, 1 out]
  n390 = String To Path(string=w29) -> (path=w16:path)
